vi "Checkers PvP No Load.vi"() -> ()   [LabVIEW 2016]
uses:
  <vilib>/Utility/miscctls.llb/LVPositionTypeDef.ctl
  Game Info Global Variable.vi
  Board Layout Global Variable.vi
panel:
  out "P2 Bottom Right Marker":picture
  out "P2 Bottom Left Marker":picture
  out "P2 Top Left Marker":picture
  out "P2 Top Right Marker":picture
  out "P1 Bottom Left Marker":picture
  out "P1 Bottom Right Marker":picture
  out "P1 Top Right Marker":picture
  out "P1 Top Left Marker":picture
  in  "Save and Quit":bool
  out "Player 2 Name":string="Player 2"
  out "Player 1 Name":string="Player 1"
  out "P2 King 12":picture
  out "P2 King 11":picture
  out "P2 King 10":picture
  out "P2 King 9":picture
  out "P2 King 8":picture
  out "P2 King 7":picture
  out "P2 King 6":picture
  out "P2 King 5":picture
  out "P2 King 4":picture
  out "P2 King 3":picture
  out "P2 King 2":picture
  out "P2 King":picture
  out "P1 King 12":picture
  out "P1 King 11":picture
  out "P1 King 10":picture
  out "P1 King 9":picture
  out "P1 King 8":picture
  out "P1 King 7":picture
  out "P1 King 6":picture
  out "P1 King 5":picture
  out "P1 King 4":picture
  out "P1 King 3":picture
  out "P1 King 2":picture
  out "P1 King":picture
  out "P2 Piece Icon":picture
  out "P1 Piece Icon":picture
  out "P2 Piece 12":picture
  out "P2 Piece 11":picture
  out "P2 Piece 10":picture
  out "P2 Piece 9":picture
  out "P2 Piece 8":picture
  out "P2 Piece 7":picture
  out "P2 Piece 6":picture
  out "P2 Piece 5":picture
  out "P2 Piece 4":picture
  out "P2 Piece 3":picture
  out "P2 Piece 2":picture
  out "P1 Piece 12":picture caption="P1 Piece"
  out "P1 Piece 11":picture caption="P1 Piece"
  out "P1 Piece 10":picture caption="P1 Piece"
  out "P1 Piece 9":picture caption="P1 Piece"
  out "P1 Piece 8":picture caption="P1 Piece"
  out "P1 Piece 7":picture caption="P1 Piece"
  out "P1 Piece 6":picture caption="P1 Piece"
  out "P1 Piece 5":picture caption="P1 Piece"
  out "P1 Piece 4":picture caption="P1 Piece"
  out "P1 Piece 3":picture caption="P1 Piece"
  out "P2 Piece":picture
  out "P1 Piece 2":picture caption="P1 Piece"
  out "Game String":string
  out "P2 Turn Light":bool
  out "P1 Turn Light":bool=TRUE
  out "P1 Piece":picture
  in  "Offer Draw":bool
  in  "Surrender":bool
  out "Player 2 Label":string="Player 1"
  out "Player 1 Label":string="Player 1"
  in  "Save":bool
  in  "Quit":bool
  # "Your Turn!"
  # "Your Turn!"
  # "678, \n308"
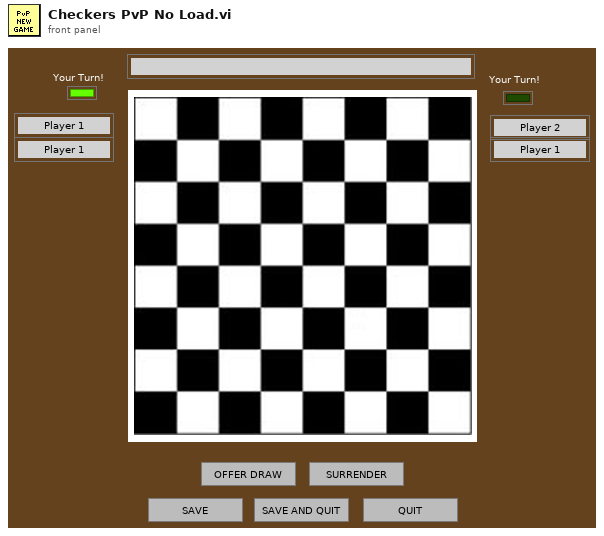
[diagram p1: front panel]
types:
  T1 = typedef "LVPositionTypeDef.ctl" = cluster{"Left":i32, "Top":i32}
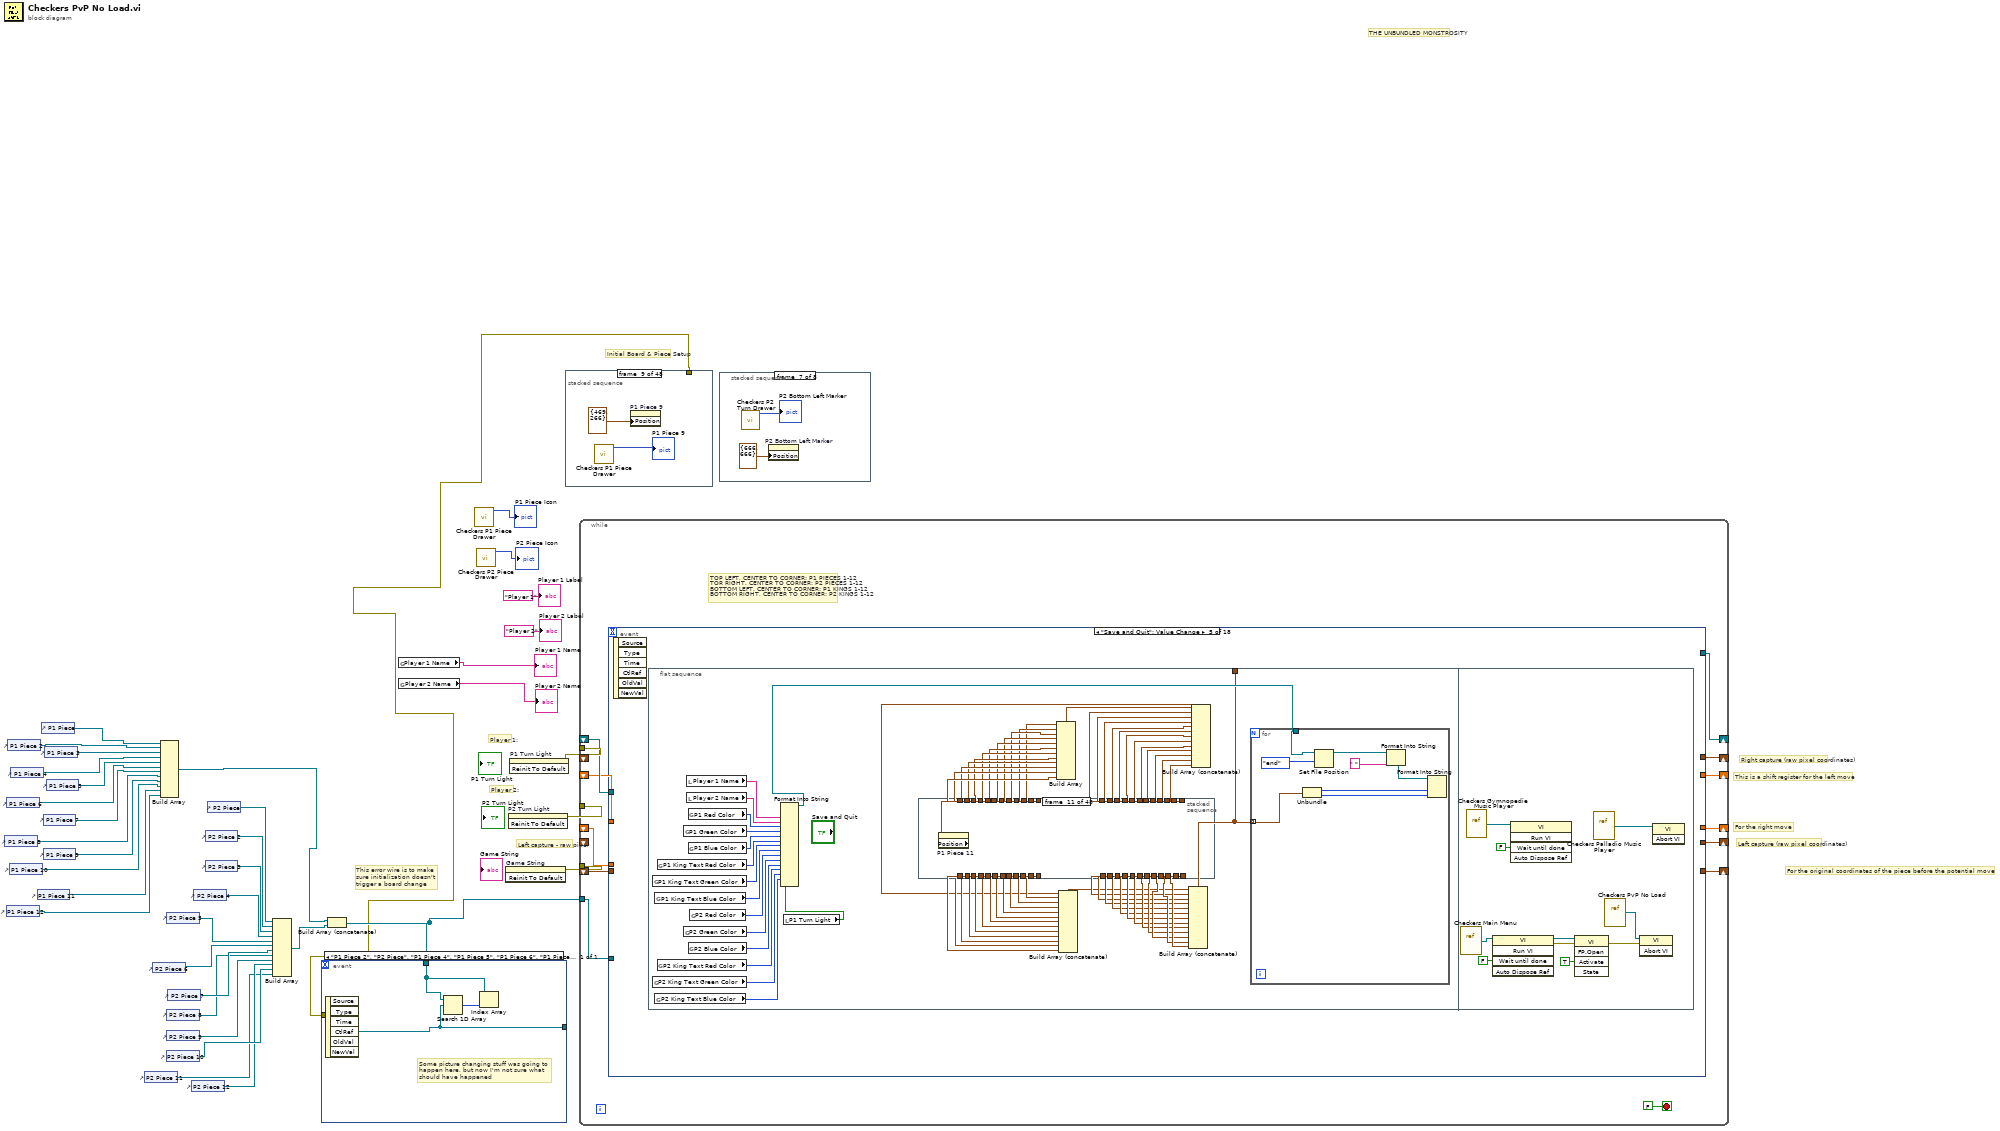
[diagram p0: block diagram]
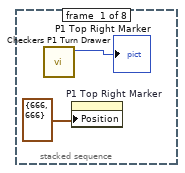
[diagram p2: hidden frame]
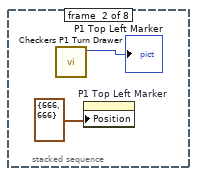
[diagram p3: hidden frame]
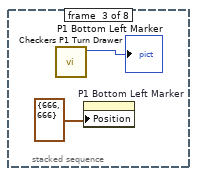
[diagram p4: hidden frame]
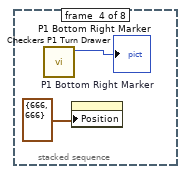
[diagram p5: hidden frame]
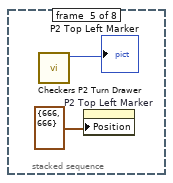
[diagram p6: hidden frame]
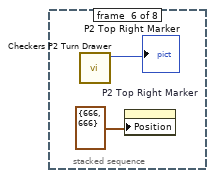
[diagram p7: hidden frame]
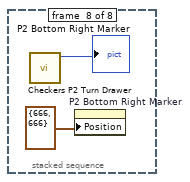
[diagram p8: hidden frame]
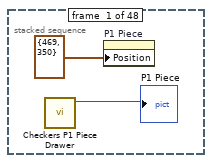
[diagram p9: hidden frame]
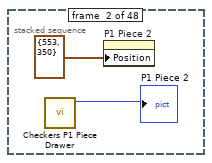
[diagram p10: hidden frame]
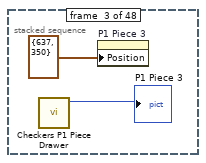
[diagram p11: hidden frame]
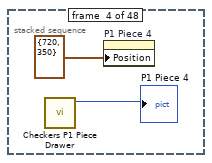
[diagram p12: hidden frame]
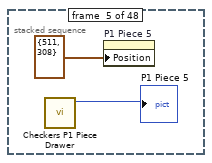
[diagram p13: hidden frame]
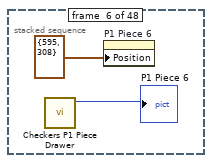
[diagram p14: hidden frame]
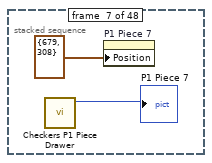
[diagram p15: hidden frame]
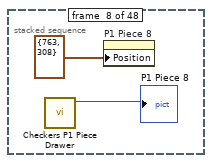
[diagram p16: hidden frame]
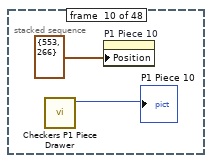
[diagram p17: hidden frame]
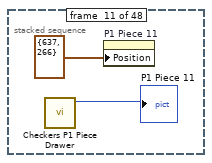
[diagram p18: hidden frame]
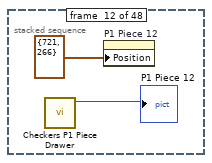
[diagram p19: hidden frame]
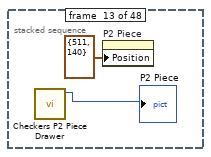
[diagram p20: hidden frame]
diagram:
  # "Left capture - raw pixel"
  # "Right capture (raw pixel coordinates)"
  # "Left capture (raw pixel coordinates)"
  # "For the original coordinates of the piece before the potential move"
  # "For the right move"
  # "This error wire is to make \nsure initialization doesn't \ntrigger a board change"
  # "This is a shift register for the left move"
  # "THE UNBUNDLED MONSTROSITY"
  # "Initial Board & Piece Setup"
  # "Player 2:"
  # "Player 1:"
  n1 = control-ref of="P1 Piece 8"() -> (w18:refnum<vi>)
  n2 = control-ref of="P1 Piece 6"() -> (w20:refnum<vi>)
  n3 = control-ref of="P1 Piece 12"() -> (w14:refnum<vi>)
  n4 = control-ref of="P1 Piece 2"() -> (w24:refnum<vi>)
  n5 = control-ref of="P1 Piece 10"() -> (w16:refnum<vi>)
  n6 = control-ref of="P1 Piece 4"() -> (w22:refnum<vi>)
  n7 = control-ref of="P1 Piece 11"() -> (w15:refnum<vi>)
  n8 = control-ref of="P1 Piece"() -> (w25:refnum<vi>)
  n9 = control-ref of="P1 Piece 7"() -> (w19:refnum<vi>)
  n10 = control-ref of="P1 Piece 9"() -> (w17:refnum<vi>)
  n11 = control-ref of="P1 Piece 3"() -> (w23:refnum<vi>)
  n12 = control-ref of="P1 Piece 5"() -> (w21:refnum<vi>)
  n13 = control-ref of="P2 Piece 11"() -> (w2:refnum<vi>)
  n14 = control-ref of="P2 Piece 6"() -> (w8:refnum<vi>)
  n15 = Build Array(w25, w24, w23, w22, w21, w20, w19, w18, w17, w16, w15, w14) -> (w1:refnum<vi>[])
  n16 = control-ref of="P2 Piece 5"() -> (w9:refnum<vi>)
  n17 = control-ref of="P2 Piece 8"() -> (w6:refnum<vi>)
  n18 = control-ref of="P2 Piece 9"() -> (w5:refnum<vi>)
  n19 = control-ref of="P2 Piece 10"() -> (w4:refnum<vi>)
  n20 = control-ref of="P2 Piece 7"() -> (w7:refnum<vi>)
  n21 = control-ref of="P2 Piece 12"() -> (w3:refnum<vi>)
  n22 = control-ref of="P2 Piece 4"() -> (w10:refnum<vi>)
  n23 = control-ref of="P2 Piece 2"() -> (w12:refnum<vi>)
  n24 = control-ref of="P2 Piece 3"() -> (w11:refnum<vi>)
  n25 = control-ref of="P2 Piece"() -> (w13:refnum<vi>)
  n26 = Build Array(w13, w12, w11, w10, w9, w8, w7, w6, w5, w3, w4, w2) -> (w29:refnum<vi>[])
  n27 = Build Array (concatenate)(w1, w29) -> (w28:refnum<vi>[])
  n28 = global read "Game Info Global Variable.vi" "Player 1 Name"() -> (→"Player 1 Name":string)
  n29 = global read "Game Info Global Variable.vi" "Player 2 Name"() -> (→"Player 2 Name":string)
  n30 = call "Checkers P1 Piece Drawer.vi"() -> ("new picture"=→"P1 Piece Icon":picture)  [unwired: 11 in]
  n31 = call "Checkers P2 Piece Drawer.vi"() -> ("new picture"=→"P2 Piece Icon":picture)  [unwired: 11 in]
  n32 = invoke on="Game String" class="Str" method="Reinit To Default"() -> (error out=w33:errorcluster)  [unwired: 3 in, 2 out]
  n33 = invoke on="P2 Turn Light" class="Bool (strict)" method="Reinit To Default"() -> (error out=w35:errorcluster)  [unwired: 3 in, 2 out]
  n34 = invoke on="P1 Turn Light" class="Bool (strict)" method="Reinit To Default"() -> (error out=w34:errorcluster)  [unwired: 3 in, 2 out]
  n35 = stacked-sequence {
    tunnel: [_ _ _ _ _ _ _ _ _ _ _ _ _ _ _ _ _ _ _ _ _ _ _ _ _ _ _ _ _ _ _ _ _ _ _ _ _ _ _ _ _ _ _ _ _ _ _ w132] -> w26
    frame #0 {
      n36 = call "Checkers P1 Piece Drawer.vi"() -> ("new picture"=→"P1 Piece":picture)  [unwired: 11 in]
      n37 = property on="P1 Piece" class="Pict"("Position"=T1 {"Left"=469, "Top"=350}) -> ()  [unwired: 2 in, 2 out]
    }
    frame #1 {
      n38 = call "Checkers P1 Piece Drawer.vi"() -> ("new picture"=→"P1 Piece 2":picture)  [unwired: 11 in]
      n39 = property on="P1 Piece 2" class="Pict"("Position"=T1 {"Left"=553, "Top"=350}) -> ()  [unwired: 2 in, 2 out]
    }
    frame #2 {
      n40 = call "Checkers P1 Piece Drawer.vi"() -> ("new picture"=→"P1 Piece 3":picture)  [unwired: 11 in]
      n41 = property on="P1 Piece 3" class="Pict"("Position"=T1 {"Left"=637, "Top"=350}) -> ()  [unwired: 2 in, 2 out]
    }
    frame #3 {
      n42 = call "Checkers P1 Piece Drawer.vi"() -> ("new picture"=→"P1 Piece 4":picture)  [unwired: 11 in]
      n43 = property on="P1 Piece 4" class="Pict"("Position"=T1 {"Left"=720, "Top"=350}) -> ()  [unwired: 2 in, 2 out]
    }
    frame #4 {
      n44 = call "Checkers P1 Piece Drawer.vi"() -> ("new picture"=→"P1 Piece 5":picture)  [unwired: 11 in]
      n45 = property on="P1 Piece 5" class="Pict"("Position"=T1 {"Left"=511, "Top"=308}) -> ()  [unwired: 2 in, 2 out]
    }
    frame #5 {
      n46 = call "Checkers P1 Piece Drawer.vi"() -> ("new picture"=→"P1 Piece 6":picture)  [unwired: 11 in]
      n47 = property on="P1 Piece 6" class="Pict"("Position"=T1 {"Left"=595, "Top"=308}) -> ()  [unwired: 2 in, 2 out]
    }
    frame #6 {
      n48 = call "Checkers P1 Piece Drawer.vi"() -> ("new picture"=→"P1 Piece 7":picture)  [unwired: 11 in]
      n49 = property on="P1 Piece 7" class="Pict"("Position"=T1 {"Left"=679, "Top"=308}) -> ()  [unwired: 2 in, 2 out]
    }
    frame #7 {
      n50 = call "Checkers P1 Piece Drawer.vi"() -> ("new picture"=→"P1 Piece 8":picture)  [unwired: 11 in]
      n51 = property on="P1 Piece 8" class="Pict"("Position"=T1 {"Left"=763, "Top"=308}) -> ()  [unwired: 2 in, 2 out]
    }
    frame #8 {
      n52 = call "Checkers P1 Piece Drawer.vi"() -> ("new picture"=→"P1 Piece 9":picture)  [unwired: 11 in]
      n53 = property on="P1 Piece 9" class="Pict"("Position"=T1 {"Left"=469, "Top"=266}) -> ()  [unwired: 2 in, 2 out]
    }
    frame #9 {
      n54 = call "Checkers P1 Piece Drawer.vi"() -> ("new picture"=→"P1 Piece 10":picture)  [unwired: 11 in]
      n55 = property on="P1 Piece 10" class="Pict"("Position"=T1 {"Left"=553, "Top"=266}) -> ()  [unwired: 2 in, 2 out]
    }
    frame #10 {
      n56 = call "Checkers P1 Piece Drawer.vi"() -> ("new picture"=→"P1 Piece 11":picture)  [unwired: 11 in]
      n57 = property on="P1 Piece 11" class="Pict"("Position"=T1 {"Left"=637, "Top"=266}) -> ()  [unwired: 2 in, 2 out]
    }
    frame #11 {
      n58 = call "Checkers P1 Piece Drawer.vi"() -> ("new picture"=→"P1 Piece 12":picture)  [unwired: 11 in]
      n59 = property on="P1 Piece 12" class="Pict"("Position"=T1 {"Left"=721, "Top"=266}) -> ()  [unwired: 2 in, 2 out]
    }
    frame #12 {
      n60 = call "Checkers P2 Piece Drawer.vi"() -> ("new picture"=→"P2 Piece":picture)  [unwired: 11 in]
      n61 = property on="P2 Piece" class="Pict"("Position"=T1 {"Left"=511, "Top"=140}) -> ()  [unwired: 2 in, 2 out]
    }
    frame #13 {
      n62 = call "Checkers P2 Piece Drawer.vi"() -> ("new picture"=→"P2 Piece 2":picture)  [unwired: 11 in]
      n63 = property on="P2 Piece 2" class="Pict"("Position"=T1 {"Left"=595, "Top"=140}) -> ()  [unwired: 2 in, 2 out]
    }
    frame #14 {
      n64 = call "Checkers P2 Piece Drawer.vi"() -> ("new picture"=→"P2 Piece 3":picture)  [unwired: 11 in]
      n65 = property on="P2 Piece 3" class="Pict"("Position"=T1 {"Left"=679, "Top"=140}) -> ()  [unwired: 2 in, 2 out]
    }
    frame #15 {
      n66 = call "Checkers P2 Piece Drawer.vi"() -> ("new picture"=→"P2 Piece 4":picture)  [unwired: 11 in]
      n67 = property on="P2 Piece 4" class="Pict"("Position"=T1 {"Left"=763, "Top"=140}) -> ()  [unwired: 2 in, 2 out]
    }
    frame #16 {
      n68 = call "Checkers P2 Piece Drawer.vi"() -> ("new picture"=→"P2 Piece 5":picture)  [unwired: 11 in]
      n69 = property on="P2 Piece 5" class="Pict"("Position"=T1 {"Left"=469, "Top"=98}) -> ()  [unwired: 2 in, 2 out]
    }
    frame #17 {
      n70 = call "Checkers P2 Piece Drawer.vi"() -> ("new picture"=→"P2 Piece 6":picture)  [unwired: 11 in]
      n71 = property on="P2 Piece 6" class="Pict"("Position"=T1 {"Left"=553, "Top"=98}) -> ()  [unwired: 2 in, 2 out]
    }
    frame #18 {
      n72 = call "Checkers P2 Piece Drawer.vi"() -> ("new picture"=→"P2 Piece 7":picture)  [unwired: 11 in]
      n73 = property on="P2 Piece 7" class="Pict"("Position"=T1 {"Left"=637, "Top"=98}) -> ()  [unwired: 2 in, 2 out]
    }
    frame #19 {
      n74 = call "Checkers P2 Piece Drawer.vi"() -> ("new picture"=→"P2 Piece 8":picture)  [unwired: 11 in]
      n75 = property on="P2 Piece 8" class="Pict"("Position"=T1 {"Left"=721, "Top"=98}) -> ()  [unwired: 2 in, 2 out]
    }
    frame #20 {
      n76 = call "Checkers P2 Piece Drawer.vi"() -> ("new picture"=→"P2 Piece 9":picture)  [unwired: 11 in]
      n77 = property on="P2 Piece 9" class="Pict"("Position"=T1 {"Left"=511, "Top"=56}) -> ()  [unwired: 2 in, 2 out]
    }
    frame #21 {
      n78 = call "Checkers P2 Piece Drawer.vi"() -> ("new picture"=→"P2 Piece 10":picture)  [unwired: 11 in]
      n79 = property on="P2 Piece 10" class="Pict"("Position"=T1 {"Left"=595, "Top"=56}) -> ()  [unwired: 2 in, 2 out]
    }
    frame #22 {
      n80 = call "Checkers P2 Piece Drawer.vi"() -> ("new picture"=→"P2 Piece 11":picture)  [unwired: 11 in]
      n81 = property on="P2 Piece 11" class="Pict"("Position"=T1 {"Left"=679, "Top"=56}) -> ()  [unwired: 2 in, 2 out]
    }
    frame #23 {
      n82 = call "Checkers P2 Piece Drawer.vi"() -> ("new picture"=→"P2 Piece 12":picture)  [unwired: 11 in]
      n83 = property on="P2 Piece 12" class="Pict"("Position"=T1 {"Left"=763, "Top"=56}) -> ()  [unwired: 2 in, 2 out]
    }
    frame #24 {
      n84 = call "Checkers P1 King Drawer.vi"() -> ("new picture"=→"P1 King":picture)  [unwired: 11 in]
      n85 = property on="P1 King" class="Pict"("Position"=T1 {"Left"=666, "Top"=666}) -> ()  [unwired: 2 in, 2 out]
    }
    frame #25 {
      n86 = call "Checkers P1 King Drawer.vi"() -> ("new picture"=→"P1 King 2":picture)  [unwired: 11 in]
      n87 = property on="P1 King 2" class="Pict"("Position"=T1 {"Left"=666, "Top"=666}) -> ()  [unwired: 2 in, 2 out]
    }
    frame #26 {
      n88 = call "Checkers P1 King Drawer.vi"() -> ("new picture"=→"P1 King 3":picture)  [unwired: 11 in]
      n89 = property on="P1 King 3" class="Pict"("Position"=T1 {"Left"=666, "Top"=666}) -> ()  [unwired: 2 in, 2 out]
    }
    frame #27 {
      n90 = call "Checkers P1 King Drawer.vi"() -> ("new picture"=→"P1 King 4":picture)  [unwired: 11 in]
      n91 = property on="P1 King 4" class="Pict"("Position"=T1 {"Left"=666, "Top"=666}) -> ()  [unwired: 2 in, 2 out]
    }
    frame #28 {
      n92 = call "Checkers P1 King Drawer.vi"() -> ("new picture"=→"P1 King 5":picture)  [unwired: 11 in]
      n93 = property on="P1 King 5" class="Pict"("Position"=T1 {"Left"=666, "Top"=666}) -> ()  [unwired: 2 in, 2 out]
    }
    frame #29 {
      n94 = call "Checkers P1 King Drawer.vi"() -> ("new picture"=→"P1 King 6":picture)  [unwired: 11 in]
      n95 = property on="P1 King 6" class="Pict"("Position"=T1 {"Left"=666, "Top"=666}) -> ()  [unwired: 2 in, 2 out]
    }
    frame #30 {
      n96 = call "Checkers P1 King Drawer.vi"() -> ("new picture"=→"P1 King 7":picture)  [unwired: 11 in]
      n97 = property on="P1 King 7" class="Pict"("Position"=T1 {"Left"=666, "Top"=666}) -> ()  [unwired: 2 in, 2 out]
    }
    frame #31 {
      n98 = call "Checkers P1 King Drawer.vi"() -> ("new picture"=→"P1 King 8":picture)  [unwired: 11 in]
      n99 = property on="P1 King 8" class="Pict"("Position"=T1 {"Left"=666, "Top"=666}) -> ()  [unwired: 2 in, 2 out]
    }
    frame #32 {
      n100 = call "Checkers P1 King Drawer.vi"() -> ("new picture"=→"P1 King 9":picture)  [unwired: 11 in]
      n101 = property on="P1 King 9" class="Pict"("Position"=T1 {"Left"=666, "Top"=666}) -> ()  [unwired: 2 in, 2 out]
    }
    frame #33 {
      n102 = call "Checkers P1 King Drawer.vi"() -> ("new picture"=→"P1 King 10":picture)  [unwired: 11 in]
      n103 = property on="P1 King 10" class="Pict"("Position"=T1 {"Left"=666, "Top"=666}) -> ()  [unwired: 2 in, 2 out]
    }
    frame #34 {
      n104 = call "Checkers P1 King Drawer.vi"() -> ("new picture"=→"P1 King 11":picture)  [unwired: 11 in]
      n105 = property on="P1 King 11" class="Pict"("Position"=T1 {"Left"=666, "Top"=666}) -> ()  [unwired: 2 in, 2 out]
    }
    frame #35 {
      n106 = call "Checkers P1 King Drawer.vi"() -> ("new picture"=→"P1 King 12":picture)  [unwired: 11 in]
      n107 = property on="P1 King 12" class="Pict"("Position"=T1 {"Left"=666, "Top"=666}) -> ()  [unwired: 2 in, 2 out]
    }
    frame #36 {
      n108 = call "Checkers P2 King Drawer.vi"() -> ("new picture"=→"P2 King":picture)  [unwired: 11 in]
      n109 = property on="P2 King" class="Pict"("Position"=T1 {"Left"=666, "Top"=666}) -> ()  [unwired: 2 in, 2 out]
    }
    frame #37 {
      n110 = call "Checkers P2 King Drawer.vi"() -> ("new picture"=→"P2 King 2":picture)  [unwired: 11 in]
      n111 = property on="P2 King 2" class="Pict"("Position"=T1 {"Left"=666, "Top"=666}) -> ()  [unwired: 2 in, 2 out]
    }
    frame #38 {
      n112 = call "Checkers P2 King Drawer.vi"() -> ("new picture"=→"P2 King 3":picture)  [unwired: 11 in]
      n113 = property on="P2 King 3" class="Pict"("Position"=T1 {"Left"=666, "Top"=666}) -> ()  [unwired: 2 in, 2 out]
    }
    frame #39 {
      n114 = call "Checkers P2 King Drawer.vi"() -> ("new picture"=→"P2 King 4":picture)  [unwired: 11 in]
      n115 = property on="P2 King 4" class="Pict"("Position"=T1 {"Left"=666, "Top"=666}) -> ()  [unwired: 2 in, 2 out]
    }
    frame #40 {
      n116 = call "Checkers P2 King Drawer.vi"() -> ("new picture"=→"P2 King 5":picture)  [unwired: 11 in]
      n117 = property on="P2 King 5" class="Pict"("Position"=T1 {"Left"=666, "Top"=666}) -> ()  [unwired: 2 in, 2 out]
    }
    frame #41 {
      n118 = call "Checkers P2 King Drawer.vi"() -> ("new picture"=→"P2 King 6":picture)  [unwired: 11 in]
      n119 = property on="P2 King 6" class="Pict"("Position"=T1 {"Left"=666, "Top"=666}) -> ()  [unwired: 2 in, 2 out]
    }
    frame #42 {
      n120 = call "Checkers P2 King Drawer.vi"() -> ("new picture"=→"P2 King 7":picture)  [unwired: 11 in]
      n121 = property on="P2 King 7" class="Pict"("Position"=T1 {"Left"=666, "Top"=666}) -> ()  [unwired: 2 in, 2 out]
    }
    frame #43 {
      n122 = call "Checkers P2 King Drawer.vi"() -> ("new picture"=→"P2 King 8":picture)  [unwired: 11 in]
      n123 = property on="P2 King 8" class="Pict"("Position"=T1 {"Left"=666, "Top"=666}) -> ()  [unwired: 2 in, 2 out]
    }
    frame #44 {
      n124 = call "Checkers P2 King Drawer.vi"() -> ("new picture"=→"P2 King 9":picture)  [unwired: 11 in]
      n125 = property on="P2 King 9" class="Pict"("Position"=T1 {"Left"=666, "Top"=666}) -> ()  [unwired: 2 in, 2 out]
    }
    frame #45 {
      n126 = call "Checkers P2 King Drawer.vi"() -> ("new picture"=→"P2 King 10":picture)  [unwired: 11 in]
      n127 = property on="P2 King 10" class="Pict"("Position"=T1 {"Left"=666, "Top"=666}) -> ()  [unwired: 2 in, 2 out]
    }
    frame #46 {
      n128 = call "Checkers P2 King Drawer.vi"() -> ("new picture"=→"P2 King 11":picture)  [unwired: 11 in]
      n129 = property on="P2 King 11" class="Pict"("Position"=T1 {"Left"=666, "Top"=666}) -> ()  [unwired: 2 in, 2 out]
    }
    frame #47 {
      n130 = call "Checkers P2 King Drawer.vi"() -> ("new picture"=→"P2 King 12":picture)  [unwired: 11 in]
      n131 = property on="P2 King 12" class="Pict"("Position"=T1 {"Left"=666, "Top"=666}) -> (error out=w132:errorcluster)  [unwired: 2 in, 1 out]
    }
  }
  n132 = event shown="[0] \"P1 Piece 2\", \"P2 Piece\", \"P1 Piece 4\", \"P1 Piece 5\", \"P1 Piece 6\", \"P1 Piece 7\", \"P1 Piece 8\", \"P1 Piece 9\", \"P1 Piece 10\", \"P1 Piece 11\", \"P1 Piece 12\", \"P2 Piece 2\", \"P2 Piece 3\", \"P2 Piece 4\", \"P2 Piece 6\", \"P2 Piece 7\", \"P2 Piece 8\", \"P2 Piece 9\", \"P2 Piece 10\", \"P2 Piece 11\", \"P2 Piece 12\": Value Change" {
    selector: _ -> [_]
    dyn-events: _ -> [_]
    timeout: _ -> [_]
    tunnel: [w137] -> _
    tunnel: w28 -> [w136]
    tunnel: w26 -> [_]
    event "P1 Piece 2", "P2 Piece", "P1 Piece 4", "P1 Piece 5", "P1 Piece 6", "P1 Piece 7", "P1 Piece 8", "P1 Piece 9", "P1 Piece 10", "P1 Piece 11", "P1 Piece 12", "P2 Piece 2", "P2 Piece 3", "P2 Piece 4", "P2 Piece 6", "P2 Piece 7", "P2 Piece 8", "P2 Piece 9", "P2 Piece 10", "P2 Piece 11", "P2 Piece 12": Value Change {
      # "Some picture changing stuff was going to \nhappen here, but now I'm not sure what \nshould have happened"
      n133 = event-data() -> ("CtlRef"=w137:refnum<vi>)  [unwired: 1 in, 5 out]
      n134 = Search 1D Array(1D array=w136, element=w137) -> (index of element=w135:i32)  [unwired: 1 in]
      n135 = Index Array(array=w136, index=w135) -> ()  [unwired: 1 out]
    }
  }
  n136 = while {
    tunnel: w35 -> [_]
    tunnel: w34 -> [_]
    tunnel: w33 -> [_]
    tunnel: w28 -> [w139]
    shift-right: [w149] -> _
    shift-left: _ -> [w148]
    shift-right: [w147] -> _
    shift-left: _ -> [w142]
    shift-right: [w146] -> _
    shift-left: _ -> [w145]
    shift-right: [w144] -> _
    shift-left: _ -> [w143]
    shift-right: [w141] -> _
    shift-left: _ -> [_]
    shift-right: [w140] -> _
    shift-left: _ -> [_]
    stop <- FALSE stop-if-true
    # "TOP LEFT, CENTER TO CORNER: P1 PIECES 1-12\nTOR RIGHT, CENTER TO CORNER: P2 PIECES 1-12\nBOTTOM LEFT, CENTER TO CORNER: P1 KINGS 1-12\nBOTTOM RIGHT, CENTER TO CORNER: P2 KINGS 1-12"
    n137 = event shown="[4] \"Save and Quit\": Value Change" {
      selector: _ -> [_ _ _ _ _ _ _ _ _ _ _ _ _ _ _ _ _ _]
      dyn-events: _ -> [_ _ _ _ _ _ _ _ _ _ _ _ _ _ _ _ _ _]
      timeout: _ -> [_ _ _ _ _ _ _ _ _ _ _ _ _ _ _ _ _ _]
      tunnel: [_ _ _ _ _ _ w527 w564 w604 w640 _ _ _ _ _ _ _ _] -> w149
      tunnel: w148 -> [_ _ _ _ _ _ _ _ _ _ w770 w781 w792 w803 w814 w829 w864 w955]
      tunnel: [_ _ _ _ _ _ w526 _ w602 _ _ _ _ _ _ _ _ _] -> w147
      tunnel: [_ _ _ _ _ _ w525 _ w603 _ _ _ _ _ _ _ _ _] -> w146
      tunnel: w145 -> [_ _ _ _ _ _ _ _ _ _ w764 _ _ _ _ _ _ _]
      tunnel: [_ _ _ _ _ _ w524 _ w600 _ _ _ _ _ _ _ _ _] -> w144
      tunnel: w143 -> [_ _ _ _ _ _ _ _ _ _ w763 _ _ _ _ w816 _ _]
      tunnel: w142 -> [_ _ _ _ _ _ _ _ _ _ _ _ _ _ _ w815 _ _]
      tunnel: [_ _ _ _ _ _ w523 _ w601 _ _ _ _ _ _ _ _ _] -> w141
      tunnel: [_ _ _ _ _ _ w522 _ _ _ _ _ _ _ _ _ _ _] -> w140
      tunnel: w139 -> [_ _ _ _ _ _ _ _ _ _ w676 _ _ _ _ _ _ _]
      event Timeout {
        n138 = event-data() -> ()  [unwired: 1 in, 3 out]
      }
      event "Offer Draw": Value Change {
        n139 = event-data() -> ()  [unwired: 1 in, 6 out]
        n140 = local read "P1 Turn Light"() -> (w150:bool)
        n141 = case shown="False" w150 {
          frame False {
            n142 = local read "Player 2 Name"() -> (w154:string)
            n143 = Format Into String(format string="%s offers a stalemate. Do you accept?", w154) -> (resulting string=w152:string)  [unwired: 2 in, 1 out]
            n144 = Two Button Dialog(message=w152, 1:"Decline" ("F button name (\"Cancel\")"), 2:"Accept" ("T button name (\"OK\")")) -> (T button?=w151:bool)
            n145 = case shown="True" w151 {
              frame False {
                # "Stalemate offer rejected. Do nothing."
              }
              frame True {
                w157 = "GAME OVER. It's a draw." ("format string")
                n146 = local write "Game String"(w157) -> ()
                n147 = Two Button Dialog(message=w157, 1:"Main Menu" ("F button name (\"Cancel\")"), 2:"New Game" ("T button name (\"OK\")")) -> (T button?=w160:bool)
                n148 = case shown="False" w160 {
                  frame False {
                    n149 = vi-ref "Checkers Main Menu.vi"() -> (w167:refnum<vi>)
                    n150 = invoke class="VI" method="Run VI"(reference=w167, "Wait until done"=FALSE ("Wait Until Done")) -> (reference out=w166:refnum<vi>, error out=w165:errorcluster)  [unwired: 3 in, 3 out]
                    n151 = invoke class="VI" method="FP.Open"(reference=w166, error in=w165, "Activate"=TRUE ("Activate?")) -> (error out=w164:errorcluster)  [unwired: 2 in, 4 out]
                    n152 = vi-ref "Checkers PvP No Load.vi"() -> (w163:refnum<vi>)
                    n153 = invoke class="VI" method="Abort VI"(reference=w163, error in=w164) -> ()  [unwired: 1 in, 3 out]
                  }
                  frame True {
                    n154 = vi-ref "Checkers New Game.vi"() -> (w174:refnum<vi>)
                    n155 = invoke class="VI" method="Run VI"(reference=w174, "Wait until done"=FALSE ("Wait Until Done")) -> (reference out=w173:refnum<vi>, error out=w172:errorcluster)  [unwired: 3 in, 3 out]
                    n156 = invoke class="VI" method="FP.Open"(reference=w173, error in=w172, "Activate"=TRUE ("Activate?")) -> (error out=w171:errorcluster)  [unwired: 2 in, 4 out]
                    n157 = vi-ref "Checkers PvP No Load.vi"() -> (w170:refnum<vi>)
                    n158 = invoke class="VI" method="Abort VI"(reference=w170, error in=w171) -> ()  [unwired: 1 in, 3 out]
                  }
                }
              }
            }
          }
          frame True {
            n159 = local read "Player 1 Name"() -> (w178:string)
            n160 = Format Into String(format string="%s offers a stalemate. Do you accept?", w178) -> (resulting string=w176:string)  [unwired: 2 in, 1 out]
            n161 = Two Button Dialog(message=w176, 1:"Decline" ("F button name (\"Cancel\")"), 2:"Accept" ("T button name (\"OK\")")) -> (T button?=w175:bool)
            n162 = case shown="True" w175 {
              frame False {
                # "Stalemate offer was rejected. Do nothing."
              }
              frame True {
                w181 = "GAME OVER. Stalemate." ("format string")
                n163 = local write "Game String"(w181) -> ()
                n164 = Two Button Dialog(message=w181, 1:"Main Menu" ("F button name (\"Cancel\")"), 2:"New Game" ("T button name (\"OK\")")) -> (T button?=w184:bool)
                n165 = case shown="False" w184 {
                  frame False {
                    n166 = vi-ref "Checkers Main Menu.vi"() -> (w191:refnum<vi>)
                    n167 = invoke class="VI" method="Run VI"(reference=w191, "Wait until done"=FALSE ("Wait Until Done")) -> (reference out=w190:refnum<vi>, error out=w189:errorcluster)  [unwired: 3 in, 3 out]
                    n168 = invoke class="VI" method="FP.Open"(reference=w190, error in=w189, "Activate"=TRUE ("Activate?")) -> (error out=w188:errorcluster)  [unwired: 2 in, 4 out]
                    n169 = vi-ref "Checkers PvP No Load.vi"() -> (w187:refnum<vi>)
                    n170 = invoke class="VI" method="Abort VI"(reference=w187, error in=w188) -> ()  [unwired: 1 in, 3 out]
                  }
                  frame True {
                    n171 = vi-ref "Checkers New Game.vi"() -> (w198:refnum<vi>)
                    n172 = invoke class="VI" method="Run VI"(reference=w198, "Wait until done"=FALSE ("Wait Until Done")) -> (reference out=w197:refnum<vi>, error out=w196:errorcluster)  [unwired: 3 in, 3 out]
                    n173 = invoke class="VI" method="FP.Open"(reference=w197, error in=w196, "Activate"=TRUE ("Activate?")) -> (error out=w195:errorcluster)  [unwired: 2 in, 4 out]
                    n174 = vi-ref "Checkers PvP No Load.vi"() -> (w194:refnum<vi>)
                    n175 = invoke class="VI" method="Abort VI"(reference=w194, error in=w195) -> ()  [unwired: 1 in, 3 out]
                  }
                }
              }
            }
          }
        }
      }
      event "Surrender": Value Change {
        n176 = event-data() -> ()  [unwired: 1 in, 6 out]
        n177 = Two Button Dialog(message="Are you sure you want to surrender?", 1:"No" ("F button name (\"Cancel\")"), 2:"Yes" ("T button name (\"OK\")")) -> (T button?=w199:bool)
        n178 = case shown="True" w199 {
          frame False {
            # "Player changed mind, didn't surrender. Do nothing."
          }
          frame True {
            n179 = local read "P1 Turn Light"() -> (w203:bool)
            n180 = case shown="True" w203 {
              frame False {
                n181 = local read "Player 1 Name"() -> (w204:string)
                n182 = Format Into String(format string="GAME OVER. %s WINS!", w204) -> (resulting string=w208:string)  [unwired: 2 in, 1 out]
                n183 = local write "Game String"(w208) -> ()
                n184 = Two Button Dialog(message=w208, 1:"Main Menu" ("F button name (\"Cancel\")"), 2:"New Game" ("T button name (\"OK\")")) -> (T button?=w205:bool)
                n185 = case shown="True" w205 {
                  frame False {
                    n186 = vi-ref "Checkers Main Menu.vi"() -> (w216:refnum<vi>)
                    n187 = invoke class="VI" method="Run VI"(reference=w216, "Wait until done"=FALSE ("Wait Until Done")) -> (reference out=w215:refnum<vi>, error out=w214:errorcluster)  [unwired: 3 in, 3 out]
                    n188 = invoke class="VI" method="FP.Open"(reference=w215, error in=w214, "Activate"=TRUE ("Activate?")) -> (error out=w213:errorcluster)  [unwired: 2 in, 4 out]
                    n189 = vi-ref "Checkers PvP No Load.vi"() -> (w212:refnum<vi>)
                    n190 = invoke class="VI" method="Abort VI"(reference=w212, error in=w213) -> ()  [unwired: 1 in, 3 out]
                  }
                  frame True {
                    n191 = vi-ref "Checkers New Game.vi"() -> (w226:refnum<vi>)
                    n192 = vi-ref "Checkers Gymnopedie Music Player.vi"() -> (w217:refnum<vi>)
                    n193 = invoke class="VI" method="Run VI"(reference=w217, "Wait until done"=FALSE ("Wait Until Done")) -> ()  [unwired: 3 in, 5 out]
                    n194 = invoke class="VI" method="Run VI"(reference=w226, "Wait until done"=FALSE ("Wait Until Done")) -> (reference out=w225:refnum<vi>, error out=w224:errorcluster)  [unwired: 3 in, 3 out]
                    n195 = vi-ref "Checkers Palladio Music Player.vi"() -> (w219:refnum<vi>)
                    n196 = invoke class="VI" method="FP.Open"(reference=w225, error in=w224, "Activate"=TRUE ("Activate?")) -> (error out=w223:errorcluster)  [unwired: 2 in, 4 out]
                    n197 = vi-ref "Checkers PvP No Load.vi"() -> (w222:refnum<vi>)
                    n198 = invoke class="VI" method="Abort VI"(reference=w219) -> ()  [unwired: 2 in, 3 out]
                    n199 = invoke class="VI" method="Abort VI"(reference=w222, error in=w223) -> ()  [unwired: 1 in, 3 out]
                  }
                }
              }
              frame True {
                n200 = local read "Player 2 Name"() -> (w227:string)
                n201 = Format Into String(format string="GAME OVER. %s WINS!", w227) -> (resulting string=w231:string)  [unwired: 2 in, 1 out]
                n202 = local write "Game String"(w231) -> ()
                n203 = Two Button Dialog(message=w231, 1:"Main Menu" ("F button name (\"Cancel\")"), 2:"New Game" ("T button name (\"OK\")")) -> (T button?=w228:bool)
                n204 = case shown="True" w228 {
                  frame False {
                    n205 = vi-ref "Checkers Main Menu.vi"() -> (w239:refnum<vi>)
                    n206 = invoke class="VI" method="Run VI"(reference=w239, "Wait until done"=FALSE ("Wait Until Done")) -> (reference out=w238:refnum<vi>, error out=w237:errorcluster)  [unwired: 3 in, 3 out]
                    n207 = invoke class="VI" method="FP.Open"(reference=w238, error in=w237, "Activate"=TRUE ("Activate?")) -> (error out=w236:errorcluster)  [unwired: 2 in, 4 out]
                    n208 = vi-ref "Checkers PvP No Load.vi"() -> (w235:refnum<vi>)
                    n209 = invoke class="VI" method="Abort VI"(reference=w235, error in=w236) -> ()  [unwired: 1 in, 3 out]
                  }
                  frame True {
                    n210 = vi-ref "Checkers New Game.vi"() -> (w249:refnum<vi>)
                    n211 = vi-ref "Checkers Gymnopedie Music Player.vi"() -> (w240:refnum<vi>)
                    n212 = invoke class="VI" method="Run VI"(reference=w249, "Wait until done"=FALSE ("Wait Until Done")) -> (reference out=w248:refnum<vi>, error out=w247:errorcluster)  [unwired: 3 in, 3 out]
                    n213 = invoke class="VI" method="Run VI"(reference=w240, "Wait until done"=FALSE ("Wait Until Done")) -> ()  [unwired: 3 in, 5 out]
                    n214 = vi-ref "Checkers Palladio Music Player.vi"() -> (w242:refnum<vi>)
                    n215 = invoke class="VI" method="FP.Open"(reference=w248, error in=w247, "Activate"=TRUE ("Activate?")) -> (error out=w246:errorcluster)  [unwired: 2 in, 4 out]
                    n216 = vi-ref "Checkers PvP No Load.vi"() -> (w245:refnum<vi>)
                    n217 = invoke class="VI" method="Abort VI"(reference=w242) -> ()  [unwired: 2 in, 3 out]
                    n218 = invoke class="VI" method="Abort VI"(reference=w245, error in=w246) -> ()  [unwired: 1 in, 3 out]
                  }
                }
              }
            }
          }
        }
      }
      event "Save": Value Change {
        n219 = event-data() -> ()  [unwired: 1 in, 6 out]
        n220 = global read "Game Info Global Variable.vi" "P1 King Text Green Color"() -> (w310:i32)
        n221 = global read "Game Info Global Variable.vi" "P2 King Text Green Color"() -> (w304:i32)
        n222 = global read "Game Info Global Variable.vi" "P1 King Text Blue Color"() -> (w309:i32)
        n223 = global read "Game Info Global Variable.vi" "P2 King Text Blue Color"() -> (w303:i32)
        n224 = global read "Game Info Global Variable.vi" "P1 King Text Red Color"() -> (w311:i32)
        n225 = global read "Game Info Global Variable.vi" "P2 King Text Red Color"() -> (w305:i32)
        n226 = local read "P1 Turn Light"() -> (w250:bool)
        n227 = global read "Game Info Global Variable.vi" "P1 Green Color"() -> (w313:i32)
        n228 = global read "Game Info Global Variable.vi" "P2 Green Color"() -> (w307:i32)
        n229 = local read "Player 1 Name"() -> (w317:string)
        n230 = local read "Player 2 Name"() -> (w316:string)
        n231 = global read "Game Info Global Variable.vi" "P1 Red Color"() -> (w314:i32)
        n232 = global read "Game Info Global Variable.vi" "P1 Blue Color"() -> (w312:i32)
        n233 = global read "Game Info Global Variable.vi" "P2 Blue Color"() -> (w306:i32)
        n234 = global read "Game Info Global Variable.vi" "P2 Red Color"() -> (w308:i32)
        n235 = Format Into String(w317, w316, w314, w313, w312, w311, w310, w309, w308, w307, w306, w305, w304, w303, w250) -> (resulting string=w315:refnum<file>)  [unwired: 3 in, 1 out]
        n236 = stacked-sequence {
          tunnel: [w318 _ _ _ _ _ _ _ _ _ _ _ _ _ _ _ _ _ _ _ _ _ _ _ _ _ _ _ _ _ _ _ _ _ _ _ _ _ _ _ _ _ _ _ _ _ _ _] -> w302
          tunnel: [_ w319 _ _ _ _ _ _ _ _ _ _ _ _ _ _ _ _ _ _ _ _ _ _ _ _ _ _ _ _ _ _ _ _ _ _ _ _ _ _ _ _ _ _ _ _ _ _] -> w301
          tunnel: [_ _ w320 _ _ _ _ _ _ _ _ _ _ _ _ _ _ _ _ _ _ _ _ _ _ _ _ _ _ _ _ _ _ _ _ _ _ _ _ _ _ _ _ _ _ _ _ _] -> w300
          tunnel: [_ _ _ w321 _ _ _ _ _ _ _ _ _ _ _ _ _ _ _ _ _ _ _ _ _ _ _ _ _ _ _ _ _ _ _ _ _ _ _ _ _ _ _ _ _ _ _ _] -> w299
          tunnel: [_ _ _ _ w322 _ _ _ _ _ _ _ _ _ _ _ _ _ _ _ _ _ _ _ _ _ _ _ _ _ _ _ _ _ _ _ _ _ _ _ _ _ _ _ _ _ _ _] -> w298
          tunnel: [_ _ _ _ _ w323 _ _ _ _ _ _ _ _ _ _ _ _ _ _ _ _ _ _ _ _ _ _ _ _ _ _ _ _ _ _ _ _ _ _ _ _ _ _ _ _ _ _] -> w297
          tunnel: [_ _ _ _ _ _ w324 _ _ _ _ _ _ _ _ _ _ _ _ _ _ _ _ _ _ _ _ _ _ _ _ _ _ _ _ _ _ _ _ _ _ _ _ _ _ _ _ _] -> w296
          tunnel: [_ _ _ _ _ _ _ w325 _ _ _ _ _ _ _ _ _ _ _ _ _ _ _ _ _ _ _ _ _ _ _ _ _ _ _ _ _ _ _ _ _ _ _ _ _ _ _ _] -> w295
          tunnel: [_ _ _ _ _ _ _ _ w326 _ _ _ _ _ _ _ _ _ _ _ _ _ _ _ _ _ _ _ _ _ _ _ _ _ _ _ _ _ _ _ _ _ _ _ _ _ _ _] -> w294
          tunnel: [_ _ _ _ _ _ _ _ _ w327 _ _ _ _ _ _ _ _ _ _ _ _ _ _ _ _ _ _ _ _ _ _ _ _ _ _ _ _ _ _ _ _ _ _ _ _ _ _] -> w293
          tunnel: [_ _ _ _ _ _ _ _ _ _ w328 _ _ _ _ _ _ _ _ _ _ _ _ _ _ _ _ _ _ _ _ _ _ _ _ _ _ _ _ _ _ _ _ _ _ _ _ _] -> w292
          tunnel: [_ _ _ _ _ _ _ _ _ _ _ w329 _ _ _ _ _ _ _ _ _ _ _ _ _ _ _ _ _ _ _ _ _ _ _ _ _ _ _ _ _ _ _ _ _ _ _ _] -> w291
          tunnel: [_ _ _ _ _ _ _ _ _ _ _ _ w330 _ _ _ _ _ _ _ _ _ _ _ _ _ _ _ _ _ _ _ _ _ _ _ _ _ _ _ _ _ _ _ _ _ _ _] -> w289
          tunnel: [_ _ _ _ _ _ _ _ _ _ _ _ _ w331 _ _ _ _ _ _ _ _ _ _ _ _ _ _ _ _ _ _ _ _ _ _ _ _ _ _ _ _ _ _ _ _ _ _] -> w288
          tunnel: [_ _ _ _ _ _ _ _ _ _ _ _ _ _ w332 _ _ _ _ _ _ _ _ _ _ _ _ _ _ _ _ _ _ _ _ _ _ _ _ _ _ _ _ _ _ _ _ _] -> w287
          tunnel: [_ _ _ _ _ _ _ _ _ _ _ _ _ _ _ w333 _ _ _ _ _ _ _ _ _ _ _ _ _ _ _ _ _ _ _ _ _ _ _ _ _ _ _ _ _ _ _ _] -> w286
          tunnel: [_ _ _ _ _ _ _ _ _ _ _ _ _ _ _ _ w334 _ _ _ _ _ _ _ _ _ _ _ _ _ _ _ _ _ _ _ _ _ _ _ _ _ _ _ _ _ _ _] -> w285
          tunnel: [_ _ _ _ _ _ _ _ _ _ _ _ _ _ _ _ _ w335 _ _ _ _ _ _ _ _ _ _ _ _ _ _ _ _ _ _ _ _ _ _ _ _ _ _ _ _ _ _] -> w284
          tunnel: [_ _ _ _ _ _ _ _ _ _ _ _ _ _ _ _ _ _ w336 _ _ _ _ _ _ _ _ _ _ _ _ _ _ _ _ _ _ _ _ _ _ _ _ _ _ _ _ _] -> w283
          tunnel: [_ _ _ _ _ _ _ _ _ _ _ _ _ _ _ _ _ _ _ w337 _ _ _ _ _ _ _ _ _ _ _ _ _ _ _ _ _ _ _ _ _ _ _ _ _ _ _ _] -> w282
          tunnel: [_ _ _ _ _ _ _ _ _ _ _ _ _ _ _ _ _ _ _ _ w338 _ _ _ _ _ _ _ _ _ _ _ _ _ _ _ _ _ _ _ _ _ _ _ _ _ _ _] -> w281
          tunnel: [_ _ _ _ _ _ _ _ _ _ _ _ _ _ _ _ _ _ _ _ _ w339 _ _ _ _ _ _ _ _ _ _ _ _ _ _ _ _ _ _ _ _ _ _ _ _ _ _] -> w280
          tunnel: [_ _ _ _ _ _ _ _ _ _ _ _ _ _ _ _ _ _ _ _ _ _ w340 _ _ _ _ _ _ _ _ _ _ _ _ _ _ _ _ _ _ _ _ _ _ _ _ _] -> w279
          tunnel: [_ _ _ _ _ _ _ _ _ _ _ _ _ _ _ _ _ _ _ _ _ _ _ w341 _ _ _ _ _ _ _ _ _ _ _ _ _ _ _ _ _ _ _ _ _ _ _ _] -> w278
          tunnel: [_ _ _ _ _ _ _ _ _ _ _ _ _ _ _ _ _ _ _ _ _ _ _ _ w342 _ _ _ _ _ _ _ _ _ _ _ _ _ _ _ _ _ _ _ _ _ _ _] -> w276
          tunnel: [_ _ _ _ _ _ _ _ _ _ _ _ _ _ _ _ _ _ _ _ _ _ _ _ _ w343 _ _ _ _ _ _ _ _ _ _ _ _ _ _ _ _ _ _ _ _ _ _] -> w275
          tunnel: [_ _ _ _ _ _ _ _ _ _ _ _ _ _ _ _ _ _ _ _ _ _ _ _ _ _ w344 _ _ _ _ _ _ _ _ _ _ _ _ _ _ _ _ _ _ _ _ _] -> w274
          tunnel: [_ _ _ _ _ _ _ _ _ _ _ _ _ _ _ _ _ _ _ _ _ _ _ _ _ _ _ w345 _ _ _ _ _ _ _ _ _ _ _ _ _ _ _ _ _ _ _ _] -> w273
          tunnel: [_ _ _ _ _ _ _ _ _ _ _ _ _ _ _ _ _ _ _ _ _ _ _ _ _ _ _ _ w346 _ _ _ _ _ _ _ _ _ _ _ _ _ _ _ _ _ _ _] -> w272
          tunnel: [_ _ _ _ _ _ _ _ _ _ _ _ _ _ _ _ _ _ _ _ _ _ _ _ _ _ _ _ _ w347 _ _ _ _ _ _ _ _ _ _ _ _ _ _ _ _ _ _] -> w271
          tunnel: [_ _ _ _ _ _ _ _ _ _ _ _ _ _ _ _ _ _ _ _ _ _ _ _ _ _ _ _ _ _ w348 _ _ _ _ _ _ _ _ _ _ _ _ _ _ _ _ _] -> w270
          tunnel: [_ _ _ _ _ _ _ _ _ _ _ _ _ _ _ _ _ _ _ _ _ _ _ _ _ _ _ _ _ _ _ w349 _ _ _ _ _ _ _ _ _ _ _ _ _ _ _ _] -> w269
          tunnel: [_ _ _ _ _ _ _ _ _ _ _ _ _ _ _ _ _ _ _ _ _ _ _ _ _ _ _ _ _ _ _ _ w350 _ _ _ _ _ _ _ _ _ _ _ _ _ _ _] -> w268
          tunnel: [_ _ _ _ _ _ _ _ _ _ _ _ _ _ _ _ _ _ _ _ _ _ _ _ _ _ _ _ _ _ _ _ _ w351 _ _ _ _ _ _ _ _ _ _ _ _ _ _] -> w267
          tunnel: [_ _ _ _ _ _ _ _ _ _ _ _ _ _ _ _ _ _ _ _ _ _ _ _ _ _ _ _ _ _ _ _ _ _ w352 _ _ _ _ _ _ _ _ _ _ _ _ _] -> w266
          tunnel: [_ _ _ _ _ _ _ _ _ _ _ _ _ _ _ _ _ _ _ _ _ _ _ _ _ _ _ _ _ _ _ _ _ _ _ w353 _ _ _ _ _ _ _ _ _ _ _ _] -> w265
          tunnel: [_ _ _ _ _ _ _ _ _ _ _ _ _ _ _ _ _ _ _ _ _ _ _ _ _ _ _ _ _ _ _ _ _ _ _ _ w354 _ _ _ _ _ _ _ _ _ _ _] -> w263
          tunnel: [_ _ _ _ _ _ _ _ _ _ _ _ _ _ _ _ _ _ _ _ _ _ _ _ _ _ _ _ _ _ _ _ _ _ _ _ _ w355 _ _ _ _ _ _ _ _ _ _] -> w262
          tunnel: [_ _ _ _ _ _ _ _ _ _ _ _ _ _ _ _ _ _ _ _ _ _ _ _ _ _ _ _ _ _ _ _ _ _ _ _ _ _ w356 _ _ _ _ _ _ _ _ _] -> w261
          tunnel: [_ _ _ _ _ _ _ _ _ _ _ _ _ _ _ _ _ _ _ _ _ _ _ _ _ _ _ _ _ _ _ _ _ _ _ _ _ _ _ w357 _ _ _ _ _ _ _ _] -> w260
          tunnel: [_ _ _ _ _ _ _ _ _ _ _ _ _ _ _ _ _ _ _ _ _ _ _ _ _ _ _ _ _ _ _ _ _ _ _ _ _ _ _ _ w358 _ _ _ _ _ _ _] -> w259
          tunnel: [_ _ _ _ _ _ _ _ _ _ _ _ _ _ _ _ _ _ _ _ _ _ _ _ _ _ _ _ _ _ _ _ _ _ _ _ _ _ _ _ _ w359 _ _ _ _ _ _] -> w258
          tunnel: [_ _ _ _ _ _ _ _ _ _ _ _ _ _ _ _ _ _ _ _ _ _ _ _ _ _ _ _ _ _ _ _ _ _ _ _ _ _ _ _ _ _ w360 _ _ _ _ _] -> w257
          tunnel: [_ _ _ _ _ _ _ _ _ _ _ _ _ _ _ _ _ _ _ _ _ _ _ _ _ _ _ _ _ _ _ _ _ _ _ _ _ _ _ _ _ _ _ w361 _ _ _ _] -> w256
          tunnel: [_ _ _ _ _ _ _ _ _ _ _ _ _ _ _ _ _ _ _ _ _ _ _ _ _ _ _ _ _ _ _ _ _ _ _ _ _ _ _ _ _ _ _ _ w362 _ _ _] -> w255
          tunnel: [_ _ _ _ _ _ _ _ _ _ _ _ _ _ _ _ _ _ _ _ _ _ _ _ _ _ _ _ _ _ _ _ _ _ _ _ _ _ _ _ _ _ _ _ _ w363 _ _] -> w254
          tunnel: [_ _ _ _ _ _ _ _ _ _ _ _ _ _ _ _ _ _ _ _ _ _ _ _ _ _ _ _ _ _ _ _ _ _ _ _ _ _ _ _ _ _ _ _ _ _ w364 _] -> w253
          tunnel: [_ _ _ _ _ _ _ _ _ _ _ _ _ _ _ _ _ _ _ _ _ _ _ _ _ _ _ _ _ _ _ _ _ _ _ _ _ _ _ _ _ _ _ _ _ _ _ w365] -> w252
          frame #0 {
            n237 = property on="P1 Piece" class="Pict"() -> ("Position"=w318:T1)  [unwired: 2 in, 2 out]
          }
          frame #1 {
            n238 = property on="P1 Piece 2" class="Pict"() -> ("Position"=w319:T1)  [unwired: 2 in, 2 out]
          }
          frame #2 {
            n239 = property on="P1 Piece 3" class="Pict"() -> ("Position"=w320:T1)  [unwired: 2 in, 2 out]
          }
          frame #3 {
            n240 = property on="P1 Piece 4" class="Pict"() -> ("Position"=w321:T1)  [unwired: 2 in, 2 out]
          }
          frame #4 {
            n241 = property on="P1 Piece 5" class="Pict"() -> ("Position"=w322:T1)  [unwired: 2 in, 2 out]
          }
          frame #5 {
            n242 = property on="P1 Piece 6" class="Pict"() -> ("Position"=w323:T1)  [unwired: 2 in, 2 out]
          }
          frame #6 {
            n243 = property on="P1 Piece 7" class="Pict"() -> ("Position"=w324:T1)  [unwired: 2 in, 2 out]
          }
          frame #7 {
            n244 = property on="P1 Piece 8" class="Pict"() -> ("Position"=w325:T1)  [unwired: 2 in, 2 out]
          }
          frame #8 {
            n245 = property on="P1 Piece 9" class="Pict"() -> ("Position"=w326:T1)  [unwired: 2 in, 2 out]
          }
          frame #9 {
            n246 = property on="P1 Piece 10" class="Pict"() -> ("Position"=w327:T1)  [unwired: 2 in, 2 out]
          }
          frame #10 {
            n247 = property on="P1 Piece 11" class="Pict"() -> ("Position"=w328:T1)  [unwired: 2 in, 2 out]
          }
          frame #11 {
            n248 = property on="P1 Piece 12" class="Pict"() -> ("Position"=w329:T1)  [unwired: 2 in, 2 out]
          }
          frame #12 {
            n249 = property on="P2 Piece" class="Pict"() -> ("Position"=w330:T1)  [unwired: 2 in, 2 out]
          }
          frame #13 {
            n250 = property on="P2 Piece 2" class="Pict"() -> ("Position"=w331:T1)  [unwired: 2 in, 2 out]
          }
          frame #14 {
            n251 = property on="P2 Piece 3" class="Pict"() -> ("Position"=w332:T1)  [unwired: 2 in, 2 out]
          }
          frame #15 {
            n252 = property on="P2 Piece 4" class="Pict"() -> ("Position"=w333:T1)  [unwired: 2 in, 2 out]
          }
          frame #16 {
            n253 = property on="P2 Piece 5" class="Pict"() -> ("Position"=w334:T1)  [unwired: 2 in, 2 out]
          }
          frame #17 {
            n254 = property on="P2 Piece 6" class="Pict"() -> ("Position"=w335:T1)  [unwired: 2 in, 2 out]
          }
          frame #18 {
            n255 = property on="P2 Piece 7" class="Pict"() -> ("Position"=w336:T1)  [unwired: 2 in, 2 out]
          }
          frame #19 {
            n256 = property on="P2 Piece 8" class="Pict"() -> ("Position"=w337:T1)  [unwired: 2 in, 2 out]
          }
          frame #20 {
            n257 = property on="P2 Piece 9" class="Pict"() -> ("Position"=w338:T1)  [unwired: 2 in, 2 out]
          }
          frame #21 {
            n258 = property on="P2 Piece 10" class="Pict"() -> ("Position"=w339:T1)  [unwired: 2 in, 2 out]
          }
          frame #22 {
            n259 = property on="P2 Piece 11" class="Pict"() -> ("Position"=w340:T1)  [unwired: 2 in, 2 out]
          }
          frame #23 {
            n260 = property on="P2 Piece 12" class="Pict"() -> ("Position"=w341:T1)  [unwired: 2 in, 2 out]
          }
          frame #24 {
            n261 = property on="P1 King" class="Pict"() -> ("Position"=w342:T1)  [unwired: 2 in, 2 out]
          }
          frame #25 {
            n262 = property on="P1 King 2" class="Pict"() -> ("Position"=w343:T1)  [unwired: 2 in, 2 out]
          }
          frame #26 {
            n263 = property on="P1 King 3" class="Pict"() -> ("Position"=w344:T1)  [unwired: 2 in, 2 out]
          }
          frame #27 {
            n264 = property on="P1 King 4" class="Pict"() -> ("Position"=w345:T1)  [unwired: 2 in, 2 out]
          }
          frame #28 {
            n265 = property on="P1 King 5" class="Pict"() -> ("Position"=w346:T1)  [unwired: 2 in, 2 out]
          }
          frame #29 {
            n266 = property on="P1 King 6" class="Pict"() -> ("Position"=w347:T1)  [unwired: 2 in, 2 out]
          }
          frame #30 {
            n267 = property on="P1 King 7" class="Pict"() -> ("Position"=w348:T1)  [unwired: 2 in, 2 out]
          }
          frame #31 {
            n268 = property on="P1 King 8" class="Pict"() -> ("Position"=w349:T1)  [unwired: 2 in, 2 out]
          }
          frame #32 {
            n269 = property on="P1 King 9" class="Pict"() -> ("Position"=w350:T1)  [unwired: 2 in, 2 out]
          }
          frame #33 {
            n270 = property on="P1 King 10" class="Pict"() -> ("Position"=w351:T1)  [unwired: 2 in, 2 out]
          }
          frame #34 {
            n271 = property on="P1 King 11" class="Pict"() -> ("Position"=w352:T1)  [unwired: 2 in, 2 out]
          }
          frame #35 {
            n272 = property on="P1 King 12" class="Pict"() -> ("Position"=w353:T1)  [unwired: 2 in, 2 out]
          }
          frame #36 {
            n273 = property on="P2 King" class="Pict"() -> ("Position"=w354:T1)  [unwired: 2 in, 2 out]
          }
          frame #37 {
            n274 = property on="P2 King 2" class="Pict"() -> ("Position"=w355:T1)  [unwired: 2 in, 2 out]
          }
          frame #38 {
            n275 = property on="P2 King 3" class="Pict"() -> ("Position"=w356:T1)  [unwired: 2 in, 2 out]
          }
          frame #39 {
            n276 = property on="P2 King 4" class="Pict"() -> ("Position"=w357:T1)  [unwired: 2 in, 2 out]
          }
          frame #40 {
            n277 = property on="P2 King 5" class="Pict"() -> ("Position"=w358:T1)  [unwired: 2 in, 2 out]
          }
          frame #41 {
            n278 = property on="P2 King 6" class="Pict"() -> ("Position"=w359:T1)  [unwired: 2 in, 2 out]
          }
          frame #42 {
            n279 = property on="P2 King 7" class="Pict"() -> ("Position"=w360:T1)  [unwired: 2 in, 2 out]
          }
          frame #43 {
            n280 = property on="P2 King 8" class="Pict"() -> ("Position"=w361:T1)  [unwired: 2 in, 2 out]
          }
          frame #44 {
            n281 = property on="P2 King 9" class="Pict"() -> ("Position"=w362:T1)  [unwired: 2 in, 2 out]
          }
          frame #45 {
            n282 = property on="P2 King 10" class="Pict"() -> ("Position"=w363:T1)  [unwired: 2 in, 2 out]
          }
          frame #46 {
            n283 = property on="P2 King 11" class="Pict"() -> ("Position"=w364:T1)  [unwired: 2 in, 2 out]
          }
          frame #47 {
            n284 = property on="P2 King 12" class="Pict"() -> ("Position"=w365:T1)  [unwired: 2 in, 2 out]
          }
        }
        n285 = Build Array(w302, w301, w300, w299, w298, w297, w296, w295, w294, w293, w292, w291) -> (w290:T1[])
        n286 = Build Array (concatenate)(w290, w289, w288, w287, w286, w285, w284, w283, w282, w281, w280, w279, w278) -> (w277:T1[])
        n287 = Build Array (concatenate)(w277, w276, w275, w274, w273, w272, w271, w270, w269, w268, w267, w266, w265) -> (w264:T1[])
        n288 = Build Array (concatenate)(w264, w263, w262, w261, w260, w259, w258, w257, w256, w255, w254, w253, w252) -> (w251:T1[])
        n289 = for {
          tunnel: w251 -> [w373] mode=indexing
          tunnel: w315 -> [w372]
          n290 = Unbundle(w373) -> ("Left"=w367:i32, "Top"=w366:i32)
          n291 = Set File Position(refnum=w372, from (0:start)=enum16{"start", "end", "current"}."end") -> (refnum out=w369:refnum<file>)  [unwired: 2 in, 1 out]
          n292 = Format Into String(initial string=w369, " " ("input 1")) -> (resulting string=w368:refnum<file>)  [unwired: 2 in, 1 out]
          n293 = Format Into String(initial string=w368, w367, w366) -> ()  [unwired: 2 in, 2 out]
        }
      }
      event "Save and Quit": Value Change {
        n294 = event-data() -> ()  [unwired: 1 in, 6 out]
        n295 = flat-sequence {
          tunnel: [w375] -> _
          frame #0 {
            n296 = global read "Game Info Global Variable.vi" "P1 King Text Green Color"() -> (w384:i32)
            n297 = global read "Game Info Global Variable.vi" "P2 King Text Green Color"() -> (w378:i32)
            n298 = global read "Game Info Global Variable.vi" "P1 King Text Blue Color"() -> (w383:i32)
            n299 = global read "Game Info Global Variable.vi" "P2 King Text Blue Color"() -> (w377:i32)
            n300 = global read "Game Info Global Variable.vi" "P1 King Text Red Color"() -> (w385:i32)
            n301 = global read "Game Info Global Variable.vi" "P2 King Text Red Color"() -> (w379:i32)
            n302 = global read "Game Info Global Variable.vi" "P1 Green Color"() -> (w387:i32)
            n303 = global read "Game Info Global Variable.vi" "P2 Green Color"() -> (w381:i32)
            n304 = local read "Player 1 Name"() -> (w390:string)
            n305 = local read "Player 2 Name"() -> (w389:string)
            n306 = global read "Game Info Global Variable.vi" "P1 Red Color"() -> (w388:i32)
            n307 = global read "Game Info Global Variable.vi" "P1 Blue Color"() -> (w386:i32)
            n308 = global read "Game Info Global Variable.vi" "P2 Blue Color"() -> (w380:i32)
            n309 = global read "Game Info Global Variable.vi" "P2 Red Color"() -> (w382:i32)
            n310 = local read "P1 Turn Light"() -> (w374:bool)
            n311 = Format Into String(w390, w389, w388, w387, w386, w385, w384, w383, w382, w381, w380, w379, w378, w377, w374) -> (resulting string=w376:refnum<file>)  [unwired: 3 in, 1 out]
            n312 = stacked-sequence {
              tunnel: [w442 _ _ _ _ _ _ _ _ _ _ _ _ _ _ _ _ _ _ _ _ _ _ _ _ _ _ _ _ _ _ _ _ _ _ _ _ _ _ _ _ _ _ _ _ _ _ _] -> w391
              tunnel: [_ w443 _ _ _ _ _ _ _ _ _ _ _ _ _ _ _ _ _ _ _ _ _ _ _ _ _ _ _ _ _ _ _ _ _ _ _ _ _ _ _ _ _ _ _ _ _ _] -> w392
              tunnel: [_ _ w444 _ _ _ _ _ _ _ _ _ _ _ _ _ _ _ _ _ _ _ _ _ _ _ _ _ _ _ _ _ _ _ _ _ _ _ _ _ _ _ _ _ _ _ _ _] -> w393
              tunnel: [_ _ _ w445 _ _ _ _ _ _ _ _ _ _ _ _ _ _ _ _ _ _ _ _ _ _ _ _ _ _ _ _ _ _ _ _ _ _ _ _ _ _ _ _ _ _ _ _] -> w394
              tunnel: [_ _ _ _ w446 _ _ _ _ _ _ _ _ _ _ _ _ _ _ _ _ _ _ _ _ _ _ _ _ _ _ _ _ _ _ _ _ _ _ _ _ _ _ _ _ _ _ _] -> w395
              tunnel: [_ _ _ _ _ w447 _ _ _ _ _ _ _ _ _ _ _ _ _ _ _ _ _ _ _ _ _ _ _ _ _ _ _ _ _ _ _ _ _ _ _ _ _ _ _ _ _ _] -> w396
              tunnel: [_ _ _ _ _ _ w448 _ _ _ _ _ _ _ _ _ _ _ _ _ _ _ _ _ _ _ _ _ _ _ _ _ _ _ _ _ _ _ _ _ _ _ _ _ _ _ _ _] -> w397
              tunnel: [_ _ _ _ _ _ _ w449 _ _ _ _ _ _ _ _ _ _ _ _ _ _ _ _ _ _ _ _ _ _ _ _ _ _ _ _ _ _ _ _ _ _ _ _ _ _ _ _] -> w398
              tunnel: [_ _ _ _ _ _ _ _ w450 _ _ _ _ _ _ _ _ _ _ _ _ _ _ _ _ _ _ _ _ _ _ _ _ _ _ _ _ _ _ _ _ _ _ _ _ _ _ _] -> w399
              tunnel: [_ _ _ _ _ _ _ _ _ w451 _ _ _ _ _ _ _ _ _ _ _ _ _ _ _ _ _ _ _ _ _ _ _ _ _ _ _ _ _ _ _ _ _ _ _ _ _ _] -> w400
              tunnel: [_ _ _ _ _ _ _ _ _ _ w452 _ _ _ _ _ _ _ _ _ _ _ _ _ _ _ _ _ _ _ _ _ _ _ _ _ _ _ _ _ _ _ _ _ _ _ _ _] -> w401
              tunnel: [_ _ _ _ _ _ _ _ _ _ _ w453 _ _ _ _ _ _ _ _ _ _ _ _ _ _ _ _ _ _ _ _ _ _ _ _ _ _ _ _ _ _ _ _ _ _ _ _] -> w402
              tunnel: [_ _ _ _ _ _ _ _ _ _ _ _ w454 _ _ _ _ _ _ _ _ _ _ _ _ _ _ _ _ _ _ _ _ _ _ _ _ _ _ _ _ _ _ _ _ _ _ _] -> w404
              tunnel: [_ _ _ _ _ _ _ _ _ _ _ _ _ w455 _ _ _ _ _ _ _ _ _ _ _ _ _ _ _ _ _ _ _ _ _ _ _ _ _ _ _ _ _ _ _ _ _ _] -> w405
              tunnel: [_ _ _ _ _ _ _ _ _ _ _ _ _ _ w456 _ _ _ _ _ _ _ _ _ _ _ _ _ _ _ _ _ _ _ _ _ _ _ _ _ _ _ _ _ _ _ _ _] -> w406
              tunnel: [_ _ _ _ _ _ _ _ _ _ _ _ _ _ _ w457 _ _ _ _ _ _ _ _ _ _ _ _ _ _ _ _ _ _ _ _ _ _ _ _ _ _ _ _ _ _ _ _] -> w407
              tunnel: [_ _ _ _ _ _ _ _ _ _ _ _ _ _ _ _ w458 _ _ _ _ _ _ _ _ _ _ _ _ _ _ _ _ _ _ _ _ _ _ _ _ _ _ _ _ _ _ _] -> w408
              tunnel: [_ _ _ _ _ _ _ _ _ _ _ _ _ _ _ _ _ w459 _ _ _ _ _ _ _ _ _ _ _ _ _ _ _ _ _ _ _ _ _ _ _ _ _ _ _ _ _ _] -> w409
              tunnel: [_ _ _ _ _ _ _ _ _ _ _ _ _ _ _ _ _ _ w460 _ _ _ _ _ _ _ _ _ _ _ _ _ _ _ _ _ _ _ _ _ _ _ _ _ _ _ _ _] -> w410
              tunnel: [_ _ _ _ _ _ _ _ _ _ _ _ _ _ _ _ _ _ _ w461 _ _ _ _ _ _ _ _ _ _ _ _ _ _ _ _ _ _ _ _ _ _ _ _ _ _ _ _] -> w411
              tunnel: [_ _ _ _ _ _ _ _ _ _ _ _ _ _ _ _ _ _ _ _ w462 _ _ _ _ _ _ _ _ _ _ _ _ _ _ _ _ _ _ _ _ _ _ _ _ _ _ _] -> w412
              tunnel: [_ _ _ _ _ _ _ _ _ _ _ _ _ _ _ _ _ _ _ _ _ w463 _ _ _ _ _ _ _ _ _ _ _ _ _ _ _ _ _ _ _ _ _ _ _ _ _ _] -> w413
              tunnel: [_ _ _ _ _ _ _ _ _ _ _ _ _ _ _ _ _ _ _ _ _ _ w464 _ _ _ _ _ _ _ _ _ _ _ _ _ _ _ _ _ _ _ _ _ _ _ _ _] -> w415
              tunnel: [_ _ _ _ _ _ _ _ _ _ _ _ _ _ _ _ _ _ _ _ _ _ _ w465 _ _ _ _ _ _ _ _ _ _ _ _ _ _ _ _ _ _ _ _ _ _ _ _] -> w414
              tunnel: [_ _ _ _ _ _ _ _ _ _ _ _ _ _ _ _ _ _ _ _ _ _ _ _ w466 _ _ _ _ _ _ _ _ _ _ _ _ _ _ _ _ _ _ _ _ _ _ _] -> w418
              tunnel: [_ _ _ _ _ _ _ _ _ _ _ _ _ _ _ _ _ _ _ _ _ _ _ _ _ w467 _ _ _ _ _ _ _ _ _ _ _ _ _ _ _ _ _ _ _ _ _ _] -> w419
              tunnel: [_ _ _ _ _ _ _ _ _ _ _ _ _ _ _ _ _ _ _ _ _ _ _ _ _ _ w468 _ _ _ _ _ _ _ _ _ _ _ _ _ _ _ _ _ _ _ _ _] -> w420
              tunnel: [_ _ _ _ _ _ _ _ _ _ _ _ _ _ _ _ _ _ _ _ _ _ _ _ _ _ _ w469 _ _ _ _ _ _ _ _ _ _ _ _ _ _ _ _ _ _ _ _] -> w421
              tunnel: [_ _ _ _ _ _ _ _ _ _ _ _ _ _ _ _ _ _ _ _ _ _ _ _ _ _ _ _ w470 _ _ _ _ _ _ _ _ _ _ _ _ _ _ _ _ _ _ _] -> w422
              tunnel: [_ _ _ _ _ _ _ _ _ _ _ _ _ _ _ _ _ _ _ _ _ _ _ _ _ _ _ _ _ w471 _ _ _ _ _ _ _ _ _ _ _ _ _ _ _ _ _ _] -> w423
              tunnel: [_ _ _ _ _ _ _ _ _ _ _ _ _ _ _ _ _ _ _ _ _ _ _ _ _ _ _ _ _ _ w472 _ _ _ _ _ _ _ _ _ _ _ _ _ _ _ _ _] -> w424
              tunnel: [_ _ _ _ _ _ _ _ _ _ _ _ _ _ _ _ _ _ _ _ _ _ _ _ _ _ _ _ _ _ _ w473 _ _ _ _ _ _ _ _ _ _ _ _ _ _ _ _] -> w425
              tunnel: [_ _ _ _ _ _ _ _ _ _ _ _ _ _ _ _ _ _ _ _ _ _ _ _ _ _ _ _ _ _ _ _ w474 _ _ _ _ _ _ _ _ _ _ _ _ _ _ _] -> w426
              tunnel: [_ _ _ _ _ _ _ _ _ _ _ _ _ _ _ _ _ _ _ _ _ _ _ _ _ _ _ _ _ _ _ _ _ w475 _ _ _ _ _ _ _ _ _ _ _ _ _ _] -> w427
              tunnel: [_ _ _ _ _ _ _ _ _ _ _ _ _ _ _ _ _ _ _ _ _ _ _ _ _ _ _ _ _ _ _ _ _ _ w476 _ _ _ _ _ _ _ _ _ _ _ _ _] -> w428
              tunnel: [_ _ _ _ _ _ _ _ _ _ _ _ _ _ _ _ _ _ _ _ _ _ _ _ _ _ _ _ _ _ _ _ _ _ _ w477 _ _ _ _ _ _ _ _ _ _ _ _] -> w429
              tunnel: [_ _ _ _ _ _ _ _ _ _ _ _ _ _ _ _ _ _ _ _ _ _ _ _ _ _ _ _ _ _ _ _ _ _ _ _ w478 _ _ _ _ _ _ _ _ _ _ _] -> w430
              tunnel: [_ _ _ _ _ _ _ _ _ _ _ _ _ _ _ _ _ _ _ _ _ _ _ _ _ _ _ _ _ _ _ _ _ _ _ _ _ w479 _ _ _ _ _ _ _ _ _ _] -> w431
              tunnel: [_ _ _ _ _ _ _ _ _ _ _ _ _ _ _ _ _ _ _ _ _ _ _ _ _ _ _ _ _ _ _ _ _ _ _ _ _ _ w480 _ _ _ _ _ _ _ _ _] -> w432
              tunnel: [_ _ _ _ _ _ _ _ _ _ _ _ _ _ _ _ _ _ _ _ _ _ _ _ _ _ _ _ _ _ _ _ _ _ _ _ _ _ _ w481 _ _ _ _ _ _ _ _] -> w433
              tunnel: [_ _ _ _ _ _ _ _ _ _ _ _ _ _ _ _ _ _ _ _ _ _ _ _ _ _ _ _ _ _ _ _ _ _ _ _ _ _ _ _ w482 _ _ _ _ _ _ _] -> w434
              tunnel: [_ _ _ _ _ _ _ _ _ _ _ _ _ _ _ _ _ _ _ _ _ _ _ _ _ _ _ _ _ _ _ _ _ _ _ _ _ _ _ _ _ w483 _ _ _ _ _ _] -> w435
              tunnel: [_ _ _ _ _ _ _ _ _ _ _ _ _ _ _ _ _ _ _ _ _ _ _ _ _ _ _ _ _ _ _ _ _ _ _ _ _ _ _ _ _ _ w484 _ _ _ _ _] -> w436
              tunnel: [_ _ _ _ _ _ _ _ _ _ _ _ _ _ _ _ _ _ _ _ _ _ _ _ _ _ _ _ _ _ _ _ _ _ _ _ _ _ _ _ _ _ _ w485 _ _ _ _] -> w437
              tunnel: [_ _ _ _ _ _ _ _ _ _ _ _ _ _ _ _ _ _ _ _ _ _ _ _ _ _ _ _ _ _ _ _ _ _ _ _ _ _ _ _ _ _ _ _ w486 _ _ _] -> w438
              tunnel: [_ _ _ _ _ _ _ _ _ _ _ _ _ _ _ _ _ _ _ _ _ _ _ _ _ _ _ _ _ _ _ _ _ _ _ _ _ _ _ _ _ _ _ _ _ w487 _ _] -> w439
              tunnel: [_ _ _ _ _ _ _ _ _ _ _ _ _ _ _ _ _ _ _ _ _ _ _ _ _ _ _ _ _ _ _ _ _ _ _ _ _ _ _ _ _ _ _ _ _ _ w488 _] -> w440
              tunnel: [_ _ _ _ _ _ _ _ _ _ _ _ _ _ _ _ _ _ _ _ _ _ _ _ _ _ _ _ _ _ _ _ _ _ _ _ _ _ _ _ _ _ _ _ _ _ _ w489] -> w441
              frame #0 {
                n313 = property on="P1 Piece" class="Pict"() -> ("Position"=w442:T1)  [unwired: 2 in, 2 out]
              }
              frame #1 {
                n314 = property on="P1 Piece 2" class="Pict"() -> ("Position"=w443:T1)  [unwired: 2 in, 2 out]
              }
              frame #2 {
                n315 = property on="P1 Piece 3" class="Pict"() -> ("Position"=w444:T1)  [unwired: 2 in, 2 out]
              }
              frame #3 {
                n316 = property on="P1 Piece 4" class="Pict"() -> ("Position"=w445:T1)  [unwired: 2 in, 2 out]
              }
              frame #4 {
                n317 = property on="P1 Piece 5" class="Pict"() -> ("Position"=w446:T1)  [unwired: 2 in, 2 out]
              }
              frame #5 {
                n318 = property on="P1 Piece 6" class="Pict"() -> ("Position"=w447:T1)  [unwired: 2 in, 2 out]
              }
              frame #6 {
                n319 = property on="P1 Piece 7" class="Pict"() -> ("Position"=w448:T1)  [unwired: 2 in, 2 out]
              }
              frame #7 {
                n320 = property on="P1 Piece 8" class="Pict"() -> ("Position"=w449:T1)  [unwired: 2 in, 2 out]
              }
              frame #8 {
                n321 = property on="P1 Piece 9" class="Pict"() -> ("Position"=w450:T1)  [unwired: 2 in, 2 out]
              }
              frame #9 {
                n322 = property on="P1 Piece 10" class="Pict"() -> ("Position"=w451:T1)  [unwired: 2 in, 2 out]
              }
              frame #10 {
                n323 = property on="P1 Piece 11" class="Pict"() -> ("Position"=w452:T1)  [unwired: 2 in, 2 out]
              }
              frame #11 {
                n324 = property on="P1 Piece 12" class="Pict"() -> ("Position"=w453:T1)  [unwired: 2 in, 2 out]
              }
              frame #12 {
                n325 = property on="P2 Piece" class="Pict"() -> ("Position"=w454:T1)  [unwired: 2 in, 2 out]
              }
              frame #13 {
                n326 = property on="P2 Piece 2" class="Pict"() -> ("Position"=w455:T1)  [unwired: 2 in, 2 out]
              }
              frame #14 {
                n327 = property on="P2 Piece 3" class="Pict"() -> ("Position"=w456:T1)  [unwired: 2 in, 2 out]
              }
              frame #15 {
                n328 = property on="P2 Piece 4" class="Pict"() -> ("Position"=w457:T1)  [unwired: 2 in, 2 out]
              }
              frame #16 {
                n329 = property on="P2 Piece 5" class="Pict"() -> ("Position"=w458:T1)  [unwired: 2 in, 2 out]
              }
              frame #17 {
                n330 = property on="P2 Piece 6" class="Pict"() -> ("Position"=w459:T1)  [unwired: 2 in, 2 out]
              }
              frame #18 {
                n331 = property on="P2 Piece 7" class="Pict"() -> ("Position"=w460:T1)  [unwired: 2 in, 2 out]
              }
              frame #19 {
                n332 = property on="P2 Piece 8" class="Pict"() -> ("Position"=w461:T1)  [unwired: 2 in, 2 out]
              }
              frame #20 {
                n333 = property on="P2 Piece 9" class="Pict"() -> ("Position"=w462:T1)  [unwired: 2 in, 2 out]
              }
              frame #21 {
                n334 = property on="P2 Piece 10" class="Pict"() -> ("Position"=w463:T1)  [unwired: 2 in, 2 out]
              }
              frame #22 {
                n335 = property on="P2 Piece 11" class="Pict"() -> ("Position"=w464:T1)  [unwired: 2 in, 2 out]
              }
              frame #23 {
                n336 = property on="P2 Piece 12" class="Pict"() -> ("Position"=w465:T1)  [unwired: 2 in, 2 out]
              }
              frame #24 {
                n337 = property on="P1 King" class="Pict"() -> ("Position"=w466:T1)  [unwired: 2 in, 2 out]
              }
              frame #25 {
                n338 = property on="P1 King 2" class="Pict"() -> ("Position"=w467:T1)  [unwired: 2 in, 2 out]
              }
              frame #26 {
                n339 = property on="P1 King 3" class="Pict"() -> ("Position"=w468:T1)  [unwired: 2 in, 2 out]
              }
              frame #27 {
                n340 = property on="P1 King 4" class="Pict"() -> ("Position"=w469:T1)  [unwired: 2 in, 2 out]
              }
              frame #28 {
                n341 = property on="P1 King 5" class="Pict"() -> ("Position"=w470:T1)  [unwired: 2 in, 2 out]
              }
              frame #29 {
                n342 = property on="P1 King 6" class="Pict"() -> ("Position"=w471:T1)  [unwired: 2 in, 2 out]
              }
              frame #30 {
                n343 = property on="P1 King 7" class="Pict"() -> ("Position"=w472:T1)  [unwired: 2 in, 2 out]
              }
              frame #31 {
                n344 = property on="P1 King 8" class="Pict"() -> ("Position"=w473:T1)  [unwired: 2 in, 2 out]
              }
              frame #32 {
                n345 = property on="P1 King 9" class="Pict"() -> ("Position"=w474:T1)  [unwired: 2 in, 2 out]
              }
              frame #33 {
                n346 = property on="P1 King 10" class="Pict"() -> ("Position"=w475:T1)  [unwired: 2 in, 2 out]
              }
              frame #34 {
                n347 = property on="P1 King 11" class="Pict"() -> ("Position"=w476:T1)  [unwired: 2 in, 2 out]
              }
              frame #35 {
                n348 = property on="P1 King 12" class="Pict"() -> ("Position"=w477:T1)  [unwired: 2 in, 2 out]
              }
              frame #36 {
                n349 = property on="P2 King" class="Pict"() -> ("Position"=w478:T1)  [unwired: 2 in, 2 out]
              }
              frame #37 {
                n350 = property on="P2 King 2" class="Pict"() -> ("Position"=w479:T1)  [unwired: 2 in, 2 out]
              }
              frame #38 {
                n351 = property on="P2 King 3" class="Pict"() -> ("Position"=w480:T1)  [unwired: 2 in, 2 out]
              }
              frame #39 {
                n352 = property on="P2 King 4" class="Pict"() -> ("Position"=w481:T1)  [unwired: 2 in, 2 out]
              }
              frame #40 {
                n353 = property on="P2 King 5" class="Pict"() -> ("Position"=w482:T1)  [unwired: 2 in, 2 out]
              }
              frame #41 {
                n354 = property on="P2 King 6" class="Pict"() -> ("Position"=w483:T1)  [unwired: 2 in, 2 out]
              }
              frame #42 {
                n355 = property on="P2 King 7" class="Pict"() -> ("Position"=w484:T1)  [unwired: 2 in, 2 out]
              }
              frame #43 {
                n356 = property on="P2 King 8" class="Pict"() -> ("Position"=w485:T1)  [unwired: 2 in, 2 out]
              }
              frame #44 {
                n357 = property on="P2 King 9" class="Pict"() -> ("Position"=w486:T1)  [unwired: 2 in, 2 out]
              }
              frame #45 {
                n358 = property on="P2 King 10" class="Pict"() -> ("Position"=w487:T1)  [unwired: 2 in, 2 out]
              }
              frame #46 {
                n359 = property on="P2 King 11" class="Pict"() -> ("Position"=w488:T1)  [unwired: 2 in, 2 out]
              }
              frame #47 {
                n360 = property on="P2 King 12" class="Pict"() -> ("Position"=w489:T1)  [unwired: 2 in, 2 out]
              }
            }
            n361 = Build Array(w391, w392, w393, w394, w395, w396, w397, w398, w399, w400, w401, w402) -> (w403:T1[])
            n362 = Build Array (concatenate)(w403, w404, w405, w406, w407, w408, w409, w410, w411, w412, w413, w415, w414) -> (w416:T1[])
            n363 = Build Array (concatenate)(w416, w418, w419, w420, w421, w422, w423, w424, w425, w426, w427, w428, w429) -> (w417:T1[])
            n364 = Build Array (concatenate)(w417, w430, w431, w432, w433, w434, w435, w436, w437, w438, w439, w440, w441) -> (w375:T1[])
            n365 = for {
              tunnel: w375 -> [w497] mode=indexing
              tunnel: w376 -> [w496]
              n366 = Unbundle(w497) -> ("Left"=w491:i32, "Top"=w490:i32)
              n367 = Set File Position(refnum=w496, from (0:start)=enum16{"start", "end", "current"}."end") -> (refnum out=w493:refnum<file>)  [unwired: 2 in, 1 out]
              n368 = Format Into String(initial string=w493, " " ("input 1")) -> (resulting string=w492:refnum<file>)  [unwired: 2 in, 1 out]
              n369 = Format Into String(initial string=w492, w491, w490) -> ()  [unwired: 2 in, 2 out]
            }
          }
          frame #1 {
            n370 = vi-ref "Checkers Main Menu.vi"() -> (w501:refnum<vi>)
            n371 = vi-ref "Checkers Gymnopedie Music Player.vi"() -> (w498:refnum<vi>)
            n372 = invoke class="VI" method="Run VI"(reference=w501, "Wait until done"=FALSE ("Wait Until Done")) -> (reference out=w502:refnum<vi>, error out=w503:errorcluster)  [unwired: 3 in, 3 out]
            n373 = invoke class="VI" method="Run VI"(reference=w498, "Wait until done"=FALSE ("Wait Until Done")) -> ()  [unwired: 3 in, 5 out]
            n374 = invoke class="VI" method="FP.Open"(reference=w502, error in=w503, "Activate"=TRUE ("Activate?")) -> (error out=w504:errorcluster)  [unwired: 2 in, 4 out]
            n375 = vi-ref "Checkers Palladio Music Player.vi"() -> (w500:refnum<vi>)
            n376 = vi-ref "Checkers PvP No Load.vi"() -> (w505:refnum<vi>)
            n377 = invoke class="VI" method="Abort VI"(reference=w505, error in=w504) -> ()  [unwired: 1 in, 3 out]
            n378 = invoke class="VI" method="Abort VI"(reference=w500) -> ()  [unwired: 2 in, 3 out]
          }
        }
      }
      event "Quit": Value Change {
        n379 = event-data() -> ()  [unwired: 1 in, 6 out]
        n380 = Two Button Dialog(message="Are you sure you want to quit without saving?", 1:"No" ("F button name (\"Cancel\")"), 2:"Yes" ("T button name (\"OK\")")) -> (T button?=w508:bool)
        n381 = case shown="False" w508 {
          frame False {
            # "Player changed mind to quit without saving. Do nothing."
          }
          frame True {
            n382 = vi-ref "Checkers Gymnopedie Music Player.vi"() -> (w512:refnum<vi>)
            n383 = vi-ref "Checkers Main Menu.vi"() -> (w521:refnum<vi>)
            n384 = invoke class="VI" method="Run VI"(reference=w521, "Wait until done"=FALSE ("Wait Until Done")) -> (reference out=w520:refnum<vi>, error out=w519:errorcluster)  [unwired: 3 in, 3 out]
            n385 = invoke class="VI" method="Run VI"(reference=w512, "Wait until done"=FALSE ("Wait Until Done")) -> ()  [unwired: 3 in, 5 out]
            n386 = invoke class="VI" method="FP.Open"(reference=w520, error in=w519, "Activate"=TRUE ("Activate?")) -> (error out=w518:errorcluster)  [unwired: 2 in, 4 out]
            n387 = vi-ref "Checkers Palladio Music Player.vi"() -> (w514:refnum<vi>)
            n388 = vi-ref "Checkers PvP No Load.vi"() -> (w517:refnum<vi>)
            n389 = invoke class="VI" method="Abort VI"(reference=w517, error in=w518) -> ()  [unwired: 1 in, 3 out]
            n390 = invoke class="VI" method="Abort VI"(reference=w514) -> ()  [unwired: 2 in, 3 out]
          }
        }
      }
      event "P1 Piece", "P1 Piece 2", "P1 Piece 3", "P1 Piece 4", "P1 Piece 5", "P1 Piece 6", "P1 Piece 7", "P1 Piece 8", "P1 Piece 9", "P1 Piece 10", "P1 Piece 11", "P1 Piece 12": Mouse Down {
        n391 = event-data() -> ("CtlRef"=w527:refnum<vi>)  [unwired: 1 in, 7 out]
        n392 = local read "P1 Turn Light"() -> (w528:bool)
        n393 = case shown="True" w528 {
          tunnel: w527 -> [_ w536]
          tunnel: [_ w533] -> w526
          tunnel: [_ w530] -> w525
          tunnel: [_ w532] -> w524
          tunnel: [_ w531] -> w523
          tunnel: [_ w529] -> w522
          frame False {
            # "It's not player 1's turn yet. Do nothing."
          }
          frame True {
            # "At this point, I use an \nequation to turn the pixel\ncoordinates into the array coordinates\nof the piece that the user clicked."
            # "Left first"
            # "row[0], collumn[1]"
            n394 = property on="Property Node" class="Pict"(reference=w536) -> ("Position"=w532:T1)  [unwired: 1 in, 2 out]
            n395 = global read "Board Layout Global Variable.vi" "Board Layout"() -> (w563:dbl[][])
            n396 = Unbundle By Name(w532) -> ("Left"=w553:i32, "Top"=w551:i32)
            n397 = expression code="(x-469)/42"(w553) -> (w554:i32)
            n398 = expression code="(x-56)/42"(w551) -> (w552:i32)
            n399 = To Long Integer(number=w554) -> (32bit integer=w537:i32)
            n400 = To Long Integer(number=w552) -> (32bit integer=w538:i32)
            n401 = Build Array(w538, w537) -> (w562:i32[])
            n402 = call "MoveLogic.vi"("Array"=w563, "Coordinates"=w562) -> ("Moves"=w559:dbl[][], "Capture 1"=w529:cluster{"Left":dbl, " Top":dbl}, "Capture 2"=w531:cluster{"Left":dbl, " Top":dbl})
            n403 = Index Array(array=w559, index (row)=0) -> (element=w533:dbl[])  [unwired: 1 in]
            n404 = Index Array(array=w559, index (row)=1) -> (element=w530:dbl[])  [unwired: 1 in]
            n405 = Index Array(array=w530, index=1) -> (element=w550:dbl)
            n406 = Index Array(array=w530, index=0) -> (element=w549:dbl)
            n407 = Index Array(array=w533, index=0) -> (element=w539:dbl)
            n408 = Index Array(array=w533, index=1) -> (element=w540:dbl)
            n409 = expression code="(x*42)+56"(w549) -> (w548:dbl)
            n410 = expression code="(x*42)+469"(w550) -> (w547:dbl)
            n411 = expression code="(x*42)+56"(w539) -> (w541:dbl)
            n412 = expression code="(x*42)+469"(w540) -> (w542:dbl)
            n413 = To Long Integer(number=w547) -> (32bit integer=w546:i32)
            n414 = To Long Integer(number=w548) -> (32bit integer=w545:i32)
            n415 = To Long Integer(number=w542) -> (32bit integer=w543:i32)
            n416 = To Long Integer(number=w541) -> (32bit integer=w544:i32)
            n417 = Bundle(w546, w545) -> (w534:cluster{i32, i32})  [unwired: 1 in]
            n418 = Bundle(w543, w544) -> (w535:cluster{i32, i32})  [unwired: 1 in]
            n419 = property on="P1 Top Right Marker" class="Pict"("Position"=w534) -> ()  [unwired: 2 in, 2 out]
            n420 = property on="P1 Top Left Marker" class="Pict"("Position"=w535) -> ()  [unwired: 2 in, 2 out]
          }
        }
      }
      event "P1 King", "P1 King 2", "P1 King 3", "P1 King 4", "P1 King 5", "P1 King 6", "P1 King 7", "P1 King 8", "P1 King 9", "P1 King 10", "P1 King 11", "P1 King 12": Mouse Down {
        n421 = event-data() -> ("CtlRef"=w564:refnum<vi>)  [unwired: 1 in, 7 out]
        n422 = local read "P1 Turn Light"() -> (w565:bool)
        n423 = case shown="True" w565 {
          tunnel: w564 -> [_ w569]
          frame False {
            # "It's not player 1's turn yet. Do nothing."
          }
          frame True {
            # "At this point, I use an \nequation to turn the pixel\ncoordinates into the array coordinates\nof the piece that the user clicked."
            # "Left first"
            # "row[0], collumn[1]"
            n424 = property on="Property Node" class="Pict"(reference=w569) -> ("Position"=w570:T1)  [unwired: 1 in, 2 out]
            n425 = global read "Board Layout Global Variable.vi" "Board Layout"() -> (w568:dbl[][])
            n426 = Unbundle By Name(w570) -> ("Left"=w590:i32, "Top"=w588:i32)
            n427 = expression code="(x-469)/42"(w590) -> (w591:i32)
            n428 = expression code="(x-56)/42"(w588) -> (w589:i32)
            n429 = To Long Integer(number=w591) -> (32bit integer=w573:i32)
            n430 = To Long Integer(number=w589) -> (32bit integer=w574:i32)
            n431 = Build Array(w574, w573) -> (w566:i32[])
            n432 = call "MoveLogic.vi"("Array"=w568, "Coordinates"=w566) -> ("Moves"=w567:dbl[][])  [unwired: 2 out]
            n433 = Index Array(array=w567, index (row)=0) -> (element=w575:dbl[])  [unwired: 1 in]
            n434 = Index Array(array=w567, index (row)=1) -> (element=w594:dbl[])  [unwired: 1 in]
            n435 = Index Array(array=w594, index=1) -> (element=w587:dbl)
            n436 = Index Array(array=w594, index=0) -> (element=w586:dbl)
            n437 = Index Array(array=w575, index=0) -> (element=w576:dbl)
            n438 = Index Array(array=w575, index=1) -> (element=w577:dbl)
            n439 = expression code="(x*42)+56"(w586) -> (w585:dbl)
            n440 = expression code="(x*42)+469"(w587) -> (w584:dbl)
            n441 = expression code="(x*42)+56"(w576) -> (w578:dbl)
            n442 = expression code="(x*42)+469"(w577) -> (w579:dbl)
            n443 = To Long Integer(number=w584) -> (32bit integer=w583:i32)
            n444 = To Long Integer(number=w585) -> (32bit integer=w582:i32)
            n445 = To Long Integer(number=w579) -> (32bit integer=w580:i32)
            n446 = To Long Integer(number=w578) -> (32bit integer=w581:i32)
            n447 = Bundle(w583, w582) -> (w572:cluster{i32, i32})  [unwired: 1 in]
            n448 = Bundle(w580, w581) -> (w571:cluster{i32, i32})  [unwired: 1 in]
            n449 = property on="P1 Top Right Marker" class="Pict"("Position"=w572) -> ()  [unwired: 2 in, 2 out]
            n450 = property on="P1 Top Left Marker" class="Pict"("Position"=w571) -> ()  [unwired: 2 in, 2 out]
          }
        }
      }
      event "P2 Piece", "P2 Piece 2", "P2 Piece 3", "P2 Piece 4", "P2 Piece 5", "P2 Piece 6", "P2 Piece 7", "P2 Piece 8", "P2 Piece 9", "P2 Piece 10", "P2 Piece 11", "P2 Piece 12": Mouse Down {
        n451 = event-data() -> ("CtlRef"=w604:refnum<vi>)  [unwired: 1 in, 7 out]
        n452 = local read "P2 Turn Light"() -> (w599:bool)
        n453 = case shown="True" w599 {
          tunnel: w604 -> [_ w614]
          tunnel: [_ w609] -> w603
          tunnel: [_ w607] -> w602
          tunnel: [_ w606] -> w601
          tunnel: [_ w605] -> w600
          frame False {
            # "It's not player 1's turn yet. Do nothing."
          }
          frame True {
            # "This sub VI outputs a 2d array \nthat holds 2 coordinates indicating \nwhere the piece can go"
            # "At this point, I use an \nequation to turn the pixel\ncoordinates into the array coordinates\nof the piece that the user clicked."
            # "Left first"
            # "row[0], collumn[1]"
            n454 = property on="Property Node" class="Pict"(reference=w614) -> ("Position"=w615:T1)  [unwired: 1 in, 2 out]
            n455 = Unbundle By Name(w615) -> ("Left"=w632:i32, "Top"=w630:i32)
            n456 = global read "Board Layout Global Variable.vi" "Board Layout"() -> (w612:dbl[][])
            n457 = expression code="(x-469)/42"(w632) -> (w633:i32)
            n458 = expression code="(x-56)/42"(w630) -> (w631:i32)
            n459 = To Long Integer(number=w633) -> (32bit integer=w616:i32)
            n460 = To Long Integer(number=w631) -> (32bit integer=w617:i32)
            n461 = Build Array(w617, w616) -> (w611:i32[])
            n462 = call "MoveLogic.vi"("Array"=w612, "Coordinates"=w611) -> ("Moves"=w610:dbl[][], "Capture 1"=w605:cluster{"Left":dbl, " Top":dbl}, "Capture 2"=w606:cluster{"Left":dbl, " Top":dbl})
            n463 = Index Array(array=w610, index (row)=0) -> (element=w609:dbl[])  [unwired: 1 in]
            n464 = Index Array(array=w610, index (row)=1) -> (element=w607:dbl[])  [unwired: 1 in]
            n465 = Index Array(array=w607, index=1) -> (element=w629:dbl)
            n466 = Index Array(array=w607, index=0) -> (element=w628:dbl)
            n467 = Index Array(array=w609, index=0) -> (element=w618:dbl)
            n468 = Index Array(array=w609, index=1) -> (element=w619:dbl)
            n469 = expression code="(x*42)+56"(w628) -> (w627:dbl)
            n470 = expression code="(x*42)+469"(w629) -> (w626:dbl)
            n471 = expression code="(x*42)+56"(w618) -> (w620:dbl)
            n472 = expression code="(x*42)+469"(w619) -> (w621:dbl)
            n473 = To Long Integer(number=w626) -> (32bit integer=w625:i32)
            n474 = To Long Integer(number=w627) -> (32bit integer=w624:i32)
            n475 = To Long Integer(number=w621) -> (32bit integer=w622:i32)
            n476 = To Long Integer(number=w620) -> (32bit integer=w623:i32)
            n477 = Bundle(w625, w624) -> (w613:cluster{i32, i32})  [unwired: 1 in]
            n478 = Bundle(w622, w623) -> (w608:cluster{i32, i32})  [unwired: 1 in]
            n479 = property on="P2 Bottom Left Marker" class="Pict"("Position"=w608) -> ()  [unwired: 2 in, 2 out]
            n480 = property on="P2 Bottom Right Marker" class="Pict"("Position"=w613) -> ()  [unwired: 2 in, 2 out]
          }
        }
      }
      event "P2 King", "P2 King 2", "P2 King 3", "P2 King 4", "P2 King 5", "P2 King 6", "P2 King 7", "P2 King 8", "P2 King 9", "P2 King 10", "P2 King 11", "P2 King 12": Mouse Down {
        n481 = event-data() -> ("CtlRef"=w640:refnum<vi>)  [unwired: 1 in, 7 out]
        n482 = local read "P2 Turn Light"() -> (w641:bool)
        n483 = case shown="True" w641 {
          tunnel: w640 -> [_ w645]
          frame False {
            # "It's not player 1's turn yet. Do nothing."
          }
          frame True {
            # "At this point, I use an \nequation to turn the pixel\ncoordinates into the array coordinates\nof the piece that the user clicked."
            # "Left first"
            # "row[0], collumn[1]"
            n484 = property on="Property Node" class="Pict"(reference=w645) -> ("Position"=w646:T1)  [unwired: 1 in, 2 out]
            n485 = global read "Board Layout Global Variable.vi" "Board Layout"() -> (w643:dbl[][])
            n486 = Unbundle By Name(w646) -> ("Left"=w666:i32, "Top"=w664:i32)
            n487 = expression code="(x-469)/42"(w666) -> (w667:i32)
            n488 = expression code="(x-56)/42"(w664) -> (w665:i32)
            n489 = To Long Integer(number=w667) -> (32bit integer=w649:i32)
            n490 = To Long Integer(number=w665) -> (32bit integer=w650:i32)
            n491 = Build Array(w650, w649) -> (w644:i32[])
            n492 = call "MoveLogic.vi"("Array"=w643, "Coordinates"=w644) -> ("Moves"=w642:dbl[][])  [unwired: 2 out]
            n493 = Index Array(array=w642, index (row)=0) -> (element=w651:dbl[])  [unwired: 1 in]
            n494 = Index Array(array=w642, index (row)=1) -> (element=w670:dbl[])  [unwired: 1 in]
            n495 = Index Array(array=w670, index=1) -> (element=w663:dbl)
            n496 = Index Array(array=w670, index=0) -> (element=w662:dbl)
            n497 = Index Array(array=w651, index=0) -> (element=w652:dbl)
            n498 = Index Array(array=w651, index=1) -> (element=w653:dbl)
            n499 = expression code="(x*42)+56"(w662) -> (w661:dbl)
            n500 = expression code="(x*42)+469"(w663) -> (w660:dbl)
            n501 = expression code="(x*42)+56"(w652) -> (w654:dbl)
            n502 = expression code="(x*42)+469"(w653) -> (w655:dbl)
            n503 = To Long Integer(number=w660) -> (32bit integer=w659:i32)
            n504 = To Long Integer(number=w661) -> (32bit integer=w658:i32)
            n505 = To Long Integer(number=w655) -> (32bit integer=w656:i32)
            n506 = To Long Integer(number=w654) -> (32bit integer=w657:i32)
            n507 = Bundle(w659, w658) -> (w648:cluster{i32, i32})  [unwired: 1 in]
            n508 = Bundle(w656, w657) -> (w647:cluster{i32, i32})  [unwired: 1 in]
            n509 = property on="P1 Top Right Marker" class="Pict"("Position"=w648) -> ()  [unwired: 2 in, 2 out]
            n510 = property on="P1 Top Left Marker" class="Pict"("Position"=w647) -> ()  [unwired: 2 in, 2 out]
          }
        }
      }
      event "P1 Top Left Marker": Mouse Down {
        n511 = event-data() -> ()  [unwired: 1 in, 8 out]
        n512 = global read "Board Layout Global Variable.vi" "Board Layout"() -> (w762:dbl[][])
        n513 = property on="P1 Top Left Marker" class="Pict"() -> (error out=w767:errorcluster, "Position"=w769:T1)  [unwired: 2 in, 1 out]
        n514 = call "FixArray.vi"("PreviousState"=w762, "Cluster"=w763, "Array 3"=w764) -> ("NewState"=w761:dbl[][])
        n515 = global write "Board Layout Global Variable.vi" "Board Layout"(w761) -> ()
        n516 = local read "P1 Turn Light"() -> (w757:bool)
        n517 = local read "P1 Turn Light"() -> (w756:bool)
        n518 = local read "P1 Turn Light"() -> (w749:bool)
        n519 = local read "P1 Turn Light"() -> (w745:bool)
        n520 = local read "P1 Turn Light"() -> (w741:bool)
        n521 = local read "P1 Turn Light"() -> (w737:bool)
        n522 = local read "P1 Turn Light"() -> (w736:bool)
        n523 = local read "P1 Turn Light"() -> (w708:bool)
        n524 = local read "P1 Turn Light"() -> (w709:bool)
        n525 = local read "P1 Turn Light"() -> (w716:bool)
        n526 = local read "P1 Turn Light"() -> (w720:bool)
        n527 = local read "P1 Turn Light"() -> (w724:bool)
        n528 = local read "P1 Turn Light"() -> (w728:bool)
        n529 = local read "P1 Turn Light"() -> (w729:bool)
        n530 = local read "P1 Turn Light"() -> (w701:bool)
        n531 = local read "P1 Turn Light"() -> (w700:bool)
        n532 = local read "P1 Turn Light"() -> (w693:bool)
        n533 = local read "P1 Turn Light"() -> (w689:bool)
        n534 = local read "P1 Turn Light"() -> (w685:bool)
        n535 = local read "P1 Turn Light"() -> (w681:bool)
        n536 = local read "P1 Turn Light"() -> (w680:bool)
        n537 = local read "P2 Turn Light"() -> (w759:bool)
        n538 = local read "P2 Turn Light"() -> (w754:bool)
        n539 = local read "P2 Turn Light"() -> (w751:bool)
        n540 = local read "P2 Turn Light"() -> (w747:bool)
        n541 = local read "P2 Turn Light"() -> (w743:bool)
        n542 = local read "P2 Turn Light"() -> (w739:bool)
        n543 = local read "P2 Turn Light"() -> (w734:bool)
        n544 = local read "P2 Turn Light"() -> (w706:bool)
        n545 = local read "P2 Turn Light"() -> (w711:bool)
        n546 = local read "P2 Turn Light"() -> (w714:bool)
        n547 = local read "P2 Turn Light"() -> (w718:bool)
        n548 = local read "P2 Turn Light"() -> (w722:bool)
        n549 = local read "P2 Turn Light"() -> (w726:bool)
        n550 = local read "P2 Turn Light"() -> (w731:bool)
        n551 = local read "P2 Turn Light"() -> (w703:bool)
        n552 = local read "P2 Turn Light"() -> (w698:bool)
        n553 = local read "P2 Turn Light"() -> (w695:bool)
        n554 = local read "P2 Turn Light"() -> (w691:bool)
        n555 = local read "P2 Turn Light"() -> (w687:bool)
        n556 = local read "P2 Turn Light"() -> (w683:bool)
        n557 = local read "P2 Turn Light"() -> (w678:bool)
        n558 = property on="Property Node" class="Pict"(reference=w770, "Position"=w769) -> ()  [unwired: 1 in, 2 out]
        n559 = Not(x=w757) -> (.not. x?=w758:bool)
        n560 = Not(x=w756) -> (.not. x?=w755:bool)
        n561 = Not(x=w749) -> (.not. x?=w750:bool)
        n562 = Not(x=w745) -> (.not. x?=w746:bool)
        n563 = Not(x=w741) -> (.not. x?=w742:bool)
        n564 = Not(x=w737) -> (.not. x?=w738:bool)
        n565 = Not(x=w736) -> (.not. x?=w735:bool)
        n566 = Not(x=w708) -> (.not. x?=w707:bool)
        n567 = Not(x=w709) -> (.not. x?=w710:bool)
        n568 = Not(x=w716) -> (.not. x?=w715:bool)
        n569 = Not(x=w720) -> (.not. x?=w719:bool)
        n570 = Not(x=w724) -> (.not. x?=w723:bool)
        n571 = Not(x=w728) -> (.not. x?=w727:bool)
        n572 = Not(x=w729) -> (.not. x?=w730:bool)
        n573 = Not(x=w701) -> (.not. x?=w702:bool)
        n574 = Not(x=w700) -> (.not. x?=w699:bool)
        n575 = Not(x=w693) -> (.not. x?=w694:bool)
        n576 = Not(x=w689) -> (.not. x?=w690:bool)
        n577 = Not(x=w685) -> (.not. x?=w686:bool)
        n578 = Not(x=w681) -> (.not. x?=w682:bool)
        n579 = Not(x=w680) -> (.not. x?=w679:bool)
        n580 = Not(x=w759) -> (.not. x?=w760:bool)
        n581 = Not(x=w754) -> (.not. x?=w753:bool)
        n582 = Not(x=w751) -> (.not. x?=w752:bool)
        n583 = Not(x=w747) -> (.not. x?=w748:bool)
        n584 = Not(x=w743) -> (.not. x?=w744:bool)
        n585 = Not(x=w739) -> (.not. x?=w740:bool)
        n586 = Not(x=w734) -> (.not. x?=w733:bool)
        n587 = Not(x=w706) -> (.not. x?=w705:bool)
        n588 = Not(x=w711) -> (.not. x?=w712:bool)
        n589 = Not(x=w714) -> (.not. x?=w713:bool)
        n590 = Not(x=w718) -> (.not. x?=w717:bool)
        n591 = Not(x=w722) -> (.not. x?=w721:bool)
        n592 = Not(x=w726) -> (.not. x?=w725:bool)
        n593 = Not(x=w731) -> (.not. x?=w732:bool)
        n594 = Not(x=w703) -> (.not. x?=w704:bool)
        n595 = Not(x=w698) -> (.not. x?=w697:bool)
        n596 = Not(x=w695) -> (.not. x?=w696:bool)
        n597 = Not(x=w691) -> (.not. x?=w692:bool)
        n598 = Not(x=w687) -> (.not. x?=w688:bool)
        n599 = Not(x=w683) -> (.not. x?=w684:bool)
        n600 = Not(x=w678) -> (.not. x?=w677:bool)
        n601 = property on="P1 Bottom Left Marker" class="Pict"("Position"=T1 {"Left"=666, "Top"=666}) -> ()  [unwired: 2 in, 2 out]
        n602 = property on="P1 Bottom Right Marker" class="Pict"("Position"=T1 {"Left"=666, "Top"=666}) -> ()  [unwired: 2 in, 2 out]
        n603 = property on="P1 Top Left Marker" class="Pict"(error in=w767, "Position"=T1 {"Left"=666, "Top"=666}) -> ()  [unwired: 1 in, 2 out]
        n604 = property on="P1 Top Right Marker" class="Pict"("Position"=T1 {"Left"=666, "Top"=666}) -> ()  [unwired: 2 in, 2 out]
        n605 = local write "P2 Turn Light"(w760) -> ()
        n606 = local write "P2 Turn Light"(w753) -> ()
        n607 = local write "P2 Turn Light"(w752) -> ()
        n608 = local write "P2 Turn Light"(w748) -> ()
        n609 = local write "P2 Turn Light"(w744) -> ()
        n610 = local write "P2 Turn Light"(w740) -> ()
        n611 = local write "P2 Turn Light"(w733) -> ()
        n612 = local write "P2 Turn Light"(w705) -> ()
        n613 = local write "P2 Turn Light"(w712) -> ()
        n614 = local write "P2 Turn Light"(w713) -> ()
        n615 = local write "P2 Turn Light"(w717) -> ()
        n616 = local write "P2 Turn Light"(w721) -> ()
        n617 = local write "P2 Turn Light"(w725) -> ()
        n618 = local write "P2 Turn Light"(w732) -> ()
        n619 = local write "P2 Turn Light"(w704) -> ()
        n620 = local write "P2 Turn Light"(w697) -> ()
        n621 = local write "P2 Turn Light"(w696) -> ()
        n622 = local write "P2 Turn Light"(w692) -> ()
        n623 = local write "P2 Turn Light"(w688) -> ()
        n624 = local write "P2 Turn Light"(w684) -> ()
        n625 = local write "P2 Turn Light"(w677) -> ()
        n626 = local write "P1 Turn Light"(w758) -> ()
        n627 = local write "P1 Turn Light"(w755) -> ()
        n628 = local write "P1 Turn Light"(w750) -> ()
        n629 = local write "P1 Turn Light"(w746) -> ()
        n630 = local write "P1 Turn Light"(w742) -> ()
        n631 = local write "P1 Turn Light"(w738) -> ()
        n632 = local write "P1 Turn Light"(w735) -> ()
        n633 = local write "P1 Turn Light"(w707) -> ()
        n634 = local write "P1 Turn Light"(w710) -> ()
        n635 = local write "P1 Turn Light"(w715) -> ()
        n636 = local write "P1 Turn Light"(w719) -> ()
        n637 = local write "P1 Turn Light"(w723) -> ()
        n638 = local write "P1 Turn Light"(w727) -> ()
        n639 = local write "P1 Turn Light"(w730) -> ()
        n640 = local write "P1 Turn Light"(w702) -> ()
        n641 = local write "P1 Turn Light"(w699) -> ()
        n642 = local write "P1 Turn Light"(w694) -> ()
        n643 = local write "P1 Turn Light"(w690) -> ()
        n644 = local write "P1 Turn Light"(w686) -> ()
        n645 = local write "P1 Turn Light"(w682) -> ()
        n646 = local write "P1 Turn Light"(w679) -> ()
        n647 = for {
          tunnel: w676 -> [_] mode=indexing
        }
      }
      event "P2 Top Left Marker": Mouse Down {
        n648 = event-data() -> ()  [unwired: 1 in, 8 out]
        n649 = property on="P2 Top Left Marker" class="Pict"() -> (error out=w778:errorcluster, "Position"=w779:T1)  [unwired: 2 in, 1 out]
        n650 = local read "P1 Turn Light"() -> (w774:bool)
        n651 = property on="Property Node" class="Pict"(reference=w781, "Position"=w779) -> ()  [unwired: 1 in, 2 out]
        n652 = local read "P2 Turn Light"() -> (w772:bool)
        n653 = Not(x=w774) -> (.not. x?=w773:bool)
        n654 = Not(x=w772) -> (.not. x?=w771:bool)
        n655 = local write "P2 Turn Light"(w771) -> ()
        n656 = property on="P2 Bottom Right Marker" class="Pict"("Position"=T1 {"Left"=666, "Top"=666}) -> ()  [unwired: 2 in, 2 out]
        n657 = property on="P2 Top Left Marker" class="Pict"(error in=w778, "Position"=T1 {"Left"=666, "Top"=666}) -> ()  [unwired: 1 in, 2 out]
        n658 = property on="P2 Top Right Marker" class="Pict"("Position"=T1 {"Left"=666, "Top"=666}) -> ()  [unwired: 2 in, 2 out]
        n659 = local write "P1 Turn Light"(w773) -> ()
        n660 = property on="P2 Bottom Left Marker" class="Pict"("Position"=T1 {"Left"=666, "Top"=666}) -> ()  [unwired: 2 in, 2 out]
      }
      event "P2 Top Right Marker": Mouse Down {
        n661 = event-data() -> ()  [unwired: 1 in, 8 out]
        n662 = property on="P2 Top Right Marker" class="Pict"() -> (error out=w786:errorcluster, "Position"=w787:T1)  [unwired: 2 in, 1 out]
        n663 = local read "P1 Turn Light"() -> (w785:bool)
        n664 = local read "P2 Turn Light"() -> (w783:bool)
        n665 = property on="Property Node" class="Pict"(reference=w792, "Position"=w787) -> ()  [unwired: 1 in, 2 out]
        n666 = Not(x=w785) -> (.not. x?=w784:bool)
        n667 = Not(x=w783) -> (.not. x?=w782:bool)
        n668 = local write "P2 Turn Light"(w782) -> ()
        n669 = local write "P1 Turn Light"(w784) -> ()
        n670 = property on="P2 Bottom Right Marker" class="Pict"("Position"=T1 {"Left"=666, "Top"=666}) -> ()  [unwired: 2 in, 2 out]
        n671 = property on="P2 Top Left Marker" class="Pict"("Position"=T1 {"Left"=666, "Top"=666}) -> ()  [unwired: 2 in, 2 out]
        n672 = property on="P2 Top Right Marker" class="Pict"(error in=w786, "Position"=T1 {"Left"=666, "Top"=666}) -> ()  [unwired: 1 in, 2 out]
        n673 = property on="P2 Bottom Left Marker" class="Pict"("Position"=T1 {"Left"=666, "Top"=666}) -> ()  [unwired: 2 in, 2 out]
      }
      event "P2 Bottom Left Marker": Mouse Down {
        n674 = event-data() -> ()  [unwired: 1 in, 8 out]
        n675 = property on="P2 Bottom Left Marker" class="Pict"() -> (error out=w797:errorcluster, "Position"=w798:T1)  [unwired: 2 in, 1 out]
        n676 = local read "P1 Turn Light"() -> (w796:bool)
        n677 = local read "P2 Turn Light"() -> (w794:bool)
        n678 = property on="Property Node" class="Pict"(reference=w803, "Position"=w798) -> ()  [unwired: 1 in, 2 out]
        n679 = Not(x=w796) -> (.not. x?=w795:bool)
        n680 = Not(x=w794) -> (.not. x?=w793:bool)
        n681 = local write "P2 Turn Light"(w793) -> ()
        n682 = local write "P1 Turn Light"(w795) -> ()
        n683 = property on="P2 Bottom Right Marker" class="Pict"("Position"=T1 {"Left"=666, "Top"=666}) -> ()  [unwired: 2 in, 2 out]
        n684 = property on="P2 Top Left Marker" class="Pict"("Position"=T1 {"Left"=666, "Top"=666}) -> ()  [unwired: 2 in, 2 out]
        n685 = property on="P2 Top Right Marker" class="Pict"("Position"=T1 {"Left"=666, "Top"=666}) -> ()  [unwired: 2 in, 2 out]
        n686 = property on="P2 Bottom Left Marker" class="Pict"(error in=w797, "Position"=T1 {"Left"=666, "Top"=666}) -> ()  [unwired: 1 in, 2 out]
      }
      event "P2 Bottom Right Marker": Mouse Down {
        n687 = event-data() -> ()  [unwired: 1 in, 8 out]
        n688 = property on="P2 Bottom Right Marker" class="Pict"() -> (error out=w808:errorcluster, "Position"=w809:T1)  [unwired: 2 in, 1 out]
        n689 = local read "P1 Turn Light"() -> (w807:bool)
        n690 = property on="Property Node" class="Pict"(reference=w814, "Position"=w809) -> ()  [unwired: 1 in, 2 out]
        n691 = local read "P2 Turn Light"() -> (w805:bool)
        n692 = Not(x=w807) -> (.not. x?=w806:bool)
        n693 = Not(x=w805) -> (.not. x?=w804:bool)
        n694 = local write "P2 Turn Light"(w804) -> ()
        n695 = property on="P2 Bottom Right Marker" class="Pict"(error in=w808, "Position"=T1 {"Left"=666, "Top"=666}) -> ()  [unwired: 1 in, 2 out]
        n696 = property on="P2 Top Left Marker" class="Pict"("Position"=T1 {"Left"=666, "Top"=666}) -> ()  [unwired: 2 in, 2 out]
        n697 = property on="P2 Top Right Marker" class="Pict"("Position"=T1 {"Left"=666, "Top"=666}) -> ()  [unwired: 2 in, 2 out]
        n698 = property on="P2 Bottom Left Marker" class="Pict"("Position"=T1 {"Left"=666, "Top"=666}) -> ()  [unwired: 2 in, 2 out]
        n699 = local write "P1 Turn Light"(w806) -> ()
      }
      event "P1 Top Right Marker": Mouse Down {
        n700 = event-data() -> ()  [unwired: 1 in, 8 out]
        n701 = property on="P1 Top Right Marker" class="Pict"() -> ("Position"=w824:T1)  [unwired: 2 in, 2 out]
        n702 = global read "Board Layout Global Variable.vi" "Board Layout"() -> (w818:dbl[][])
        n703 = call "FixArray.vi"("PreviousState"=w818, "Cluster"=w816, "Array 3"=w815) -> ("NewState"=w817:dbl[][])
        n704 = global write "Board Layout Global Variable.vi" "Board Layout"(w817) -> ()
        n705 = property on="Property Node" class="Pict"(reference=w829, "Position"=w824) -> (error out=w823:errorcluster)  [unwired: 1 in, 1 out]
        n706 = property on="P1 Bottom Left Marker" class="Pict"("Position"=T1 {"Left"=666, "Top"=666}) -> ()  [unwired: 2 in, 2 out]
        n707 = property on="P1 Bottom Right Marker" class="Pict"("Position"=T1 {"Left"=666, "Top"=666}) -> ()  [unwired: 2 in, 2 out]
        n708 = property on="P1 Top Left Marker" class="Pict"("Position"=T1 {"Left"=666, "Top"=666}) -> ()  [unwired: 2 in, 2 out]
        n709 = property on="P1 Top Right Marker" class="Pict"(error in=w823, "Position"=T1 {"Left"=666, "Top"=666}) -> ()  [unwired: 1 in, 2 out]
        n710 = local read "P1 Turn Light"() -> (w822:bool)
        n711 = local read "P2 Turn Light"() -> (w820:bool)
        n712 = Not(x=w822) -> (.not. x?=w821:bool)
        n713 = Not(x=w820) -> (.not. x?=w819:bool)
        n714 = local write "P2 Turn Light"(w819) -> ()
        n715 = local write "P1 Turn Light"(w821) -> ()
      }
      event "P1 Bottom Left Marker": Mouse Down {
        n716 = event-data() -> ()  [unwired: 1 in, 8 out]
        n717 = property on="P1 Bottom Left Marker" class="Pict"() -> ("Position"=w859:T1)  [unwired: 2 in, 2 out]
        n718 = local read "P1 Turn Light"() -> (w854:bool)
        n719 = local read "P1 Turn Light"() -> (w853:bool)
        n720 = local read "P1 Turn Light"() -> (w846:bool)
        n721 = local read "P1 Turn Light"() -> (w842:bool)
        n722 = local read "P1 Turn Light"() -> (w838:bool)
        n723 = local read "P1 Turn Light"() -> (w834:bool)
        n724 = local read "P1 Turn Light"() -> (w833:bool)
        n725 = local read "P2 Turn Light"() -> (w856:bool)
        n726 = local read "P2 Turn Light"() -> (w851:bool)
        n727 = local read "P2 Turn Light"() -> (w848:bool)
        n728 = local read "P2 Turn Light"() -> (w844:bool)
        n729 = local read "P2 Turn Light"() -> (w840:bool)
        n730 = local read "P2 Turn Light"() -> (w836:bool)
        n731 = local read "P2 Turn Light"() -> (w831:bool)
        n732 = property on="Property Node" class="Pict"(reference=w864, "Position"=w859) -> (error out=w858:errorcluster)  [unwired: 1 in, 1 out]
        n733 = Not(x=w854) -> (.not. x?=w855:bool)
        n734 = Not(x=w853) -> (.not. x?=w852:bool)
        n735 = Not(x=w846) -> (.not. x?=w847:bool)
        n736 = Not(x=w842) -> (.not. x?=w843:bool)
        n737 = Not(x=w838) -> (.not. x?=w839:bool)
        n738 = Not(x=w834) -> (.not. x?=w835:bool)
        n739 = Not(x=w833) -> (.not. x?=w832:bool)
        n740 = Not(x=w856) -> (.not. x?=w857:bool)
        n741 = Not(x=w851) -> (.not. x?=w850:bool)
        n742 = Not(x=w848) -> (.not. x?=w849:bool)
        n743 = Not(x=w844) -> (.not. x?=w845:bool)
        n744 = Not(x=w840) -> (.not. x?=w841:bool)
        n745 = Not(x=w836) -> (.not. x?=w837:bool)
        n746 = Not(x=w831) -> (.not. x?=w830:bool)
        n747 = local write "P2 Turn Light"(w857) -> ()
        n748 = local write "P2 Turn Light"(w850) -> ()
        n749 = local write "P2 Turn Light"(w849) -> ()
        n750 = local write "P2 Turn Light"(w845) -> ()
        n751 = local write "P2 Turn Light"(w841) -> ()
        n752 = local write "P2 Turn Light"(w837) -> ()
        n753 = local write "P2 Turn Light"(w830) -> ()
        n754 = local write "P1 Turn Light"(w855) -> ()
        n755 = local write "P1 Turn Light"(w852) -> ()
        n756 = local write "P1 Turn Light"(w847) -> ()
        n757 = local write "P1 Turn Light"(w843) -> ()
        n758 = local write "P1 Turn Light"(w839) -> ()
        n759 = local write "P1 Turn Light"(w835) -> ()
        n760 = local write "P1 Turn Light"(w832) -> ()
        n761 = property on="P1 Bottom Left Marker" class="Pict"(error in=w858, "Position"=T1 {"Left"=666, "Top"=666}) -> ()  [unwired: 1 in, 2 out]
        n762 = property on="P1 Bottom Right Marker" class="Pict"("Position"=T1 {"Left"=666, "Top"=666}) -> ()  [unwired: 2 in, 2 out]
        n763 = property on="P1 Top Left Marker" class="Pict"("Position"=T1 {"Left"=666, "Top"=666}) -> ()  [unwired: 2 in, 2 out]
        n764 = property on="P1 Top Right Marker" class="Pict"("Position"=T1 {"Left"=666, "Top"=666}) -> ()  [unwired: 2 in, 2 out]
      }
      event "P1 Bottom Right Marker": Mouse Down {
        n765 = event-data() -> ()  [unwired: 1 in, 8 out]
        n766 = property on="P1 Bottom Right Marker" class="Pict"() -> ("Position"=w950:T1)  [unwired: 2 in, 2 out]
        n767 = local read "P1 Turn Light"() -> (w945:bool)
        n768 = local read "P1 Turn Light"() -> (w944:bool)
        n769 = local read "P1 Turn Light"() -> (w937:bool)
        n770 = local read "P1 Turn Light"() -> (w933:bool)
        n771 = local read "P1 Turn Light"() -> (w929:bool)
        n772 = local read "P1 Turn Light"() -> (w925:bool)
        n773 = local read "P1 Turn Light"() -> (w924:bool)
        n774 = local read "P1 Turn Light"() -> (w896:bool)
        n775 = local read "P1 Turn Light"() -> (w897:bool)
        n776 = local read "P1 Turn Light"() -> (w904:bool)
        n777 = local read "P1 Turn Light"() -> (w908:bool)
        n778 = local read "P1 Turn Light"() -> (w912:bool)
        n779 = local read "P1 Turn Light"() -> (w916:bool)
        n780 = local read "P1 Turn Light"() -> (w917:bool)
        n781 = local read "P1 Turn Light"() -> (w889:bool)
        n782 = local read "P1 Turn Light"() -> (w888:bool)
        n783 = local read "P1 Turn Light"() -> (w881:bool)
        n784 = local read "P1 Turn Light"() -> (w877:bool)
        n785 = local read "P1 Turn Light"() -> (w873:bool)
        n786 = local read "P1 Turn Light"() -> (w869:bool)
        n787 = local read "P1 Turn Light"() -> (w868:bool)
        n788 = local read "P2 Turn Light"() -> (w947:bool)
        n789 = local read "P2 Turn Light"() -> (w942:bool)
        n790 = local read "P2 Turn Light"() -> (w939:bool)
        n791 = local read "P2 Turn Light"() -> (w935:bool)
        n792 = local read "P2 Turn Light"() -> (w931:bool)
        n793 = local read "P2 Turn Light"() -> (w927:bool)
        n794 = local read "P2 Turn Light"() -> (w922:bool)
        n795 = local read "P2 Turn Light"() -> (w894:bool)
        n796 = local read "P2 Turn Light"() -> (w899:bool)
        n797 = local read "P2 Turn Light"() -> (w902:bool)
        n798 = local read "P2 Turn Light"() -> (w906:bool)
        n799 = local read "P2 Turn Light"() -> (w910:bool)
        n800 = local read "P2 Turn Light"() -> (w914:bool)
        n801 = local read "P2 Turn Light"() -> (w919:bool)
        n802 = local read "P2 Turn Light"() -> (w891:bool)
        n803 = local read "P2 Turn Light"() -> (w886:bool)
        n804 = local read "P2 Turn Light"() -> (w883:bool)
        n805 = local read "P2 Turn Light"() -> (w879:bool)
        n806 = local read "P2 Turn Light"() -> (w875:bool)
        n807 = local read "P2 Turn Light"() -> (w871:bool)
        n808 = local read "P2 Turn Light"() -> (w866:bool)
        n809 = property on="Property Node" class="Pict"(reference=w955, "Position"=w950) -> (error out=w949:errorcluster)  [unwired: 1 in, 1 out]
        n810 = Not(x=w945) -> (.not. x?=w946:bool)
        n811 = Not(x=w944) -> (.not. x?=w943:bool)
        n812 = Not(x=w937) -> (.not. x?=w938:bool)
        n813 = Not(x=w933) -> (.not. x?=w934:bool)
        n814 = Not(x=w929) -> (.not. x?=w930:bool)
        n815 = Not(x=w925) -> (.not. x?=w926:bool)
        n816 = Not(x=w924) -> (.not. x?=w923:bool)
        n817 = Not(x=w896) -> (.not. x?=w895:bool)
        n818 = Not(x=w897) -> (.not. x?=w898:bool)
        n819 = Not(x=w904) -> (.not. x?=w903:bool)
        n820 = Not(x=w908) -> (.not. x?=w907:bool)
        n821 = Not(x=w912) -> (.not. x?=w911:bool)
        n822 = Not(x=w916) -> (.not. x?=w915:bool)
        n823 = Not(x=w917) -> (.not. x?=w918:bool)
        n824 = Not(x=w889) -> (.not. x?=w890:bool)
        n825 = Not(x=w888) -> (.not. x?=w887:bool)
        n826 = Not(x=w881) -> (.not. x?=w882:bool)
        n827 = Not(x=w877) -> (.not. x?=w878:bool)
        n828 = Not(x=w873) -> (.not. x?=w874:bool)
        n829 = Not(x=w869) -> (.not. x?=w870:bool)
        n830 = Not(x=w868) -> (.not. x?=w867:bool)
        n831 = Not(x=w947) -> (.not. x?=w948:bool)
        n832 = Not(x=w942) -> (.not. x?=w941:bool)
        n833 = Not(x=w939) -> (.not. x?=w940:bool)
        n834 = Not(x=w935) -> (.not. x?=w936:bool)
        n835 = Not(x=w931) -> (.not. x?=w932:bool)
        n836 = Not(x=w927) -> (.not. x?=w928:bool)
        n837 = Not(x=w922) -> (.not. x?=w921:bool)
        n838 = Not(x=w894) -> (.not. x?=w893:bool)
        n839 = Not(x=w899) -> (.not. x?=w900:bool)
        n840 = Not(x=w902) -> (.not. x?=w901:bool)
        n841 = Not(x=w906) -> (.not. x?=w905:bool)
        n842 = Not(x=w910) -> (.not. x?=w909:bool)
        n843 = Not(x=w914) -> (.not. x?=w913:bool)
        n844 = Not(x=w919) -> (.not. x?=w920:bool)
        n845 = Not(x=w891) -> (.not. x?=w892:bool)
        n846 = Not(x=w886) -> (.not. x?=w885:bool)
        n847 = Not(x=w883) -> (.not. x?=w884:bool)
        n848 = Not(x=w879) -> (.not. x?=w880:bool)
        n849 = Not(x=w875) -> (.not. x?=w876:bool)
        n850 = Not(x=w871) -> (.not. x?=w872:bool)
        n851 = Not(x=w866) -> (.not. x?=w865:bool)
        n852 = local write "P2 Turn Light"(w948) -> ()
        n853 = local write "P2 Turn Light"(w941) -> ()
        n854 = local write "P2 Turn Light"(w940) -> ()
        n855 = local write "P2 Turn Light"(w936) -> ()
        n856 = local write "P2 Turn Light"(w932) -> ()
        n857 = local write "P2 Turn Light"(w928) -> ()
        n858 = local write "P2 Turn Light"(w921) -> ()
        n859 = local write "P2 Turn Light"(w893) -> ()
        n860 = local write "P2 Turn Light"(w900) -> ()
        n861 = local write "P2 Turn Light"(w901) -> ()
        n862 = local write "P2 Turn Light"(w905) -> ()
        n863 = local write "P2 Turn Light"(w909) -> ()
        n864 = local write "P2 Turn Light"(w913) -> ()
        n865 = local write "P2 Turn Light"(w920) -> ()
        n866 = local write "P2 Turn Light"(w892) -> ()
        n867 = local write "P2 Turn Light"(w885) -> ()
        n868 = local write "P2 Turn Light"(w884) -> ()
        n869 = local write "P2 Turn Light"(w880) -> ()
        n870 = local write "P2 Turn Light"(w876) -> ()
        n871 = local write "P2 Turn Light"(w872) -> ()
        n872 = local write "P2 Turn Light"(w865) -> ()
        n873 = local write "P1 Turn Light"(w946) -> ()
        n874 = local write "P1 Turn Light"(w943) -> ()
        n875 = local write "P1 Turn Light"(w938) -> ()
        n876 = local write "P1 Turn Light"(w934) -> ()
        n877 = local write "P1 Turn Light"(w930) -> ()
        n878 = local write "P1 Turn Light"(w926) -> ()
        n879 = local write "P1 Turn Light"(w923) -> ()
        n880 = local write "P1 Turn Light"(w895) -> ()
        n881 = local write "P1 Turn Light"(w898) -> ()
        n882 = local write "P1 Turn Light"(w903) -> ()
        n883 = local write "P1 Turn Light"(w907) -> ()
        n884 = local write "P1 Turn Light"(w911) -> ()
        n885 = local write "P1 Turn Light"(w915) -> ()
        n886 = local write "P1 Turn Light"(w918) -> ()
        n887 = local write "P1 Turn Light"(w890) -> ()
        n888 = local write "P1 Turn Light"(w887) -> ()
        n889 = local write "P1 Turn Light"(w882) -> ()
        n890 = local write "P1 Turn Light"(w878) -> ()
        n891 = local write "P1 Turn Light"(w874) -> ()
        n892 = local write "P1 Turn Light"(w870) -> ()
        n893 = local write "P1 Turn Light"(w867) -> ()
        n894 = property on="P1 Top Left Marker" class="Pict"("Position"=T1 {"Left"=666, "Top"=666}) -> ()  [unwired: 2 in, 2 out]
        n895 = property on="P1 Top Right Marker" class="Pict"("Position"=T1 {"Left"=666, "Top"=666}) -> ()  [unwired: 2 in, 2 out]
        n896 = property on="P1 Bottom Right Marker" class="Pict"(error in=w949, "Position"=T1 {"Left"=666, "Top"=666}) -> ()  [unwired: 1 in, 2 out]
        n897 = property on="P1 Bottom Left Marker" class="Pict"("Position"=T1 {"Left"=666, "Top"=666}) -> ()  [unwired: 2 in, 2 out]
      }
    }
  }
  n898 = stacked-sequence {
    frame #0 {
      n899 = call "Checkers P1 Turn Drawer.vi"() -> ("new picture"=→"P1 Top Right Marker":picture)  [unwired: 11 in]
      n900 = property on="P1 Top Right Marker" class="Pict"("Position"=T1 {"Left"=666, "Top"=666}) -> ()  [unwired: 2 in, 2 out]
    }
    frame #1 {
      n901 = call "Checkers P1 Turn Drawer.vi"() -> ("new picture"=→"P1 Top Left Marker":picture)  [unwired: 11 in]
      n902 = property on="P1 Top Left Marker" class="Pict"("Position"=T1 {"Left"=666, "Top"=666}) -> ()  [unwired: 2 in, 2 out]
    }
    frame #2 {
      n903 = call "Checkers P1 Turn Drawer.vi"() -> ("new picture"=→"P1 Bottom Left Marker":picture)  [unwired: 11 in]
      n904 = property on="P1 Bottom Left Marker" class="Pict"("Position"=T1 {"Left"=666, "Top"=666}) -> ()  [unwired: 2 in, 2 out]
    }
    frame #3 {
      n905 = call "Checkers P1 Turn Drawer.vi"() -> ("new picture"=→"P1 Bottom Right Marker":picture)  [unwired: 11 in]
      n906 = property on="P1 Bottom Right Marker" class="Pict"("Position"=T1 {"Left"=666, "Top"=666}) -> ()  [unwired: 2 in, 2 out]
    }
    frame #4 {
      n907 = call "Checkers P2 Turn Drawer.vi"() -> ("new picture"=→"P2 Top Left Marker":picture)  [unwired: 11 in]
      n908 = property on="P2 Top Left Marker" class="Pict"("Position"=T1 {"Left"=666, "Top"=666}) -> ()  [unwired: 2 in, 2 out]
    }
    frame #5 {
      n909 = call "Checkers P2 Turn Drawer.vi"() -> ("new picture"=→"P2 Top Right Marker":picture)  [unwired: 11 in]
      n910 = property on="P2 Top Right Marker" class="Pict"("Position"=T1 {"Left"=666, "Top"=666}) -> ()  [unwired: 2 in, 2 out]
    }
    frame #6 {
      n911 = call "Checkers P2 Turn Drawer.vi"() -> ("new picture"=→"P2 Bottom Left Marker":picture)  [unwired: 11 in]
      n912 = property on="P2 Bottom Left Marker" class="Pict"("Position"=T1 {"Left"=666, "Top"=666}) -> ()  [unwired: 2 in, 2 out]
    }
    frame #7 {
      n913 = call "Checkers P2 Turn Drawer.vi"() -> ("new picture"=→"P2 Bottom Right Marker":picture)  [unwired: 11 in]
      n914 = property on="P2 Bottom Right Marker" class="Pict"("Position"=T1 {"Left"=666, "Top"=666}) -> ()  [unwired: 2 in, 2 out]
    }
  }
  "Player 1 Label" <- "Player 1" ("String 3")
  "Player 2 Label" <- "Player 2" ("String 4")
